vi "8255-led .vi"() -> ()   [LabVIEW 2010]
uses:
  <vilib>/LabVIEW Interface for Arduino/Type Defs/Pin Mode.ctl
  <vilib>/LabVIEW Interface for Arduino/LabVIEW Interface for Arduino.lvlib
panel:
  in  "Boolean":bool
  in  "OK Button":bool
  in  "Slide":dbl(slide) scale=0.0..1.0
  in  "stop":bool
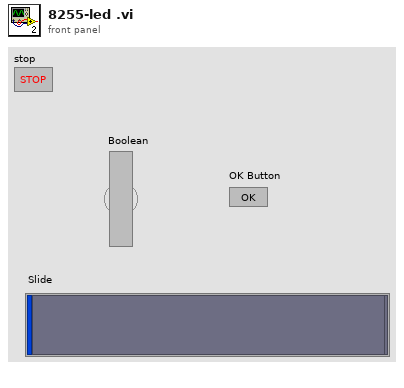
[diagram p1: front panel]
types:
  T1 = typedef "LabVIEW Interface for Arduino.lvlib/Arduino Resource.ctl" = cluster{"VISA resource":refnum<visa-resource-name>, "Board Type":T2, "Connection Type":enum8{"USB / Serial"}, "Bytes Per Packet (15)":u8}
  T2 = typedef "LabVIEW Interface for Arduino.lvlib/Board Type.ctl" = enum16{"Uno", "Dimuelanove w/Atmega 328", "Mega 2560"}
  T3 = typedef "LabVIEW Interface for Arduino.lvlib/Pin Mode.ctl" = enum8{"Input", "Output"}
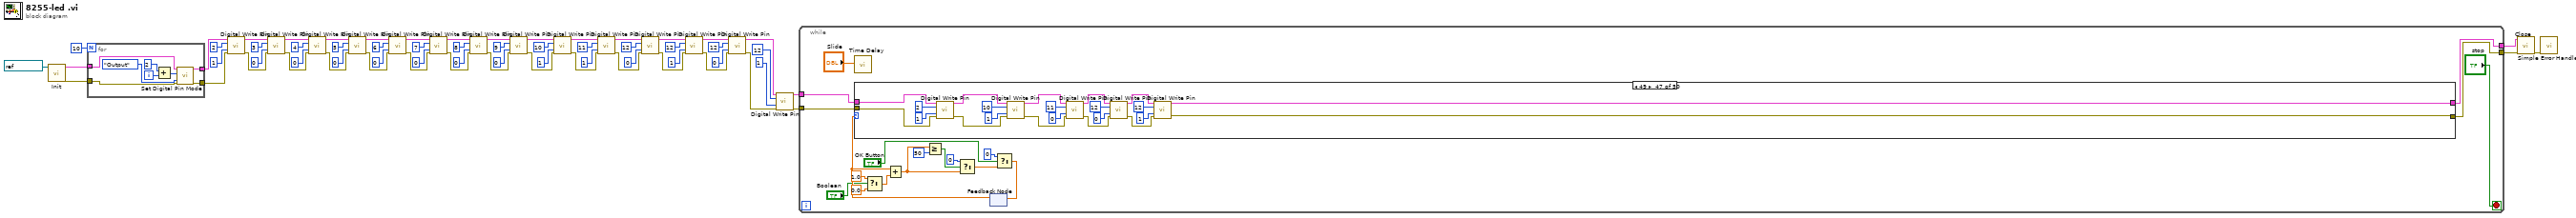
[diagram p0: block diagram]
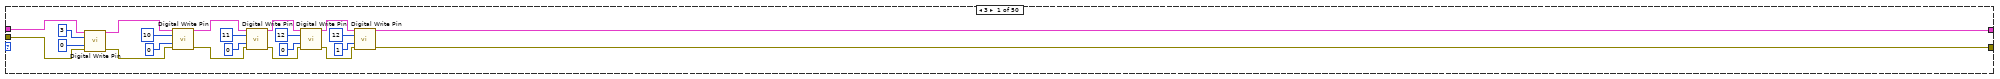
[diagram p2: hidden frame]
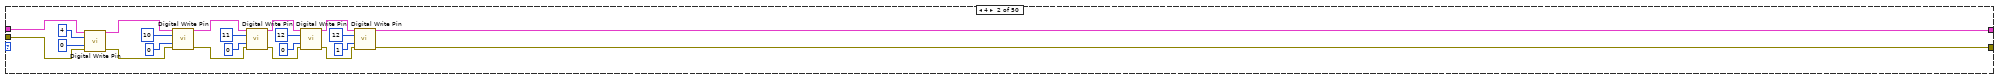
[diagram p3: hidden frame]
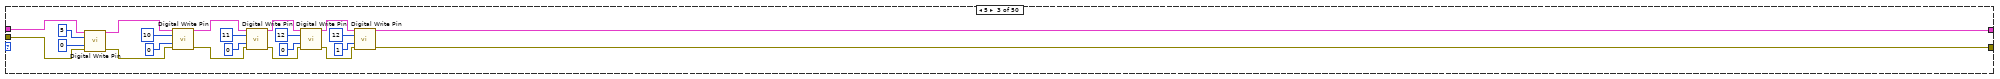
[diagram p4: hidden frame]
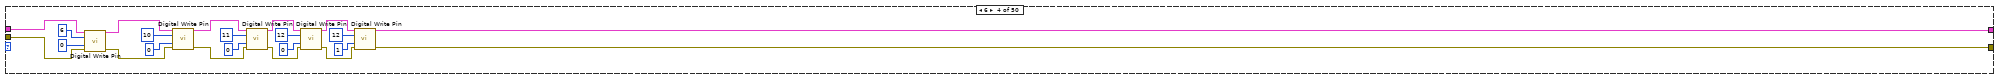
[diagram p5: hidden frame]
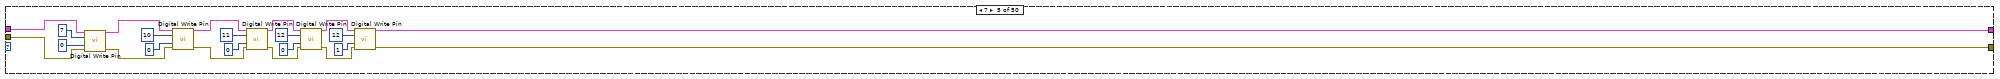
[diagram p6: hidden frame]
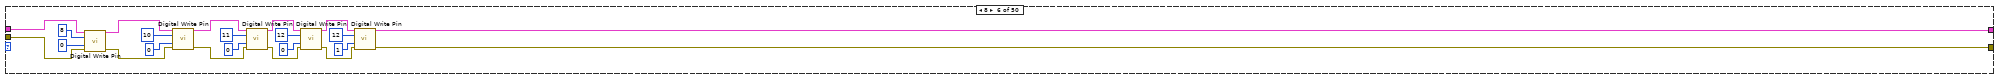
[diagram p7: hidden frame]
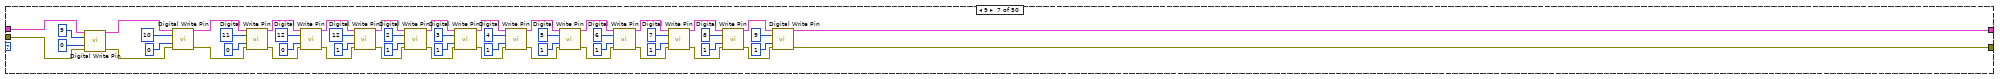
[diagram p8: hidden frame]
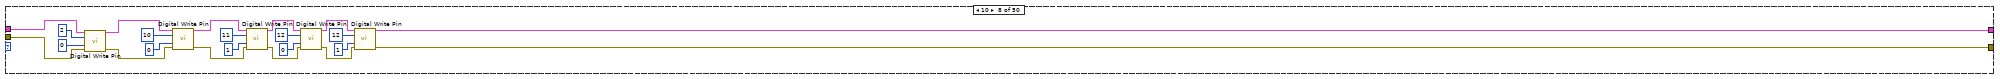
[diagram p9: hidden frame]
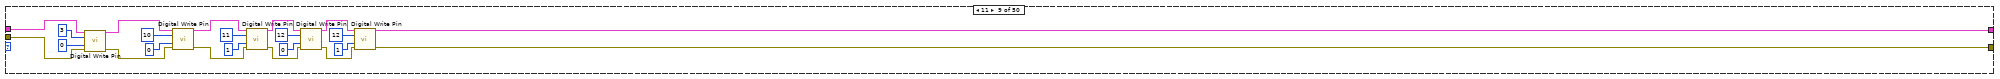
[diagram p10: hidden frame]
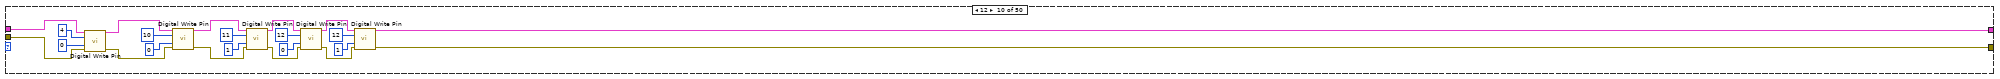
[diagram p11: hidden frame]
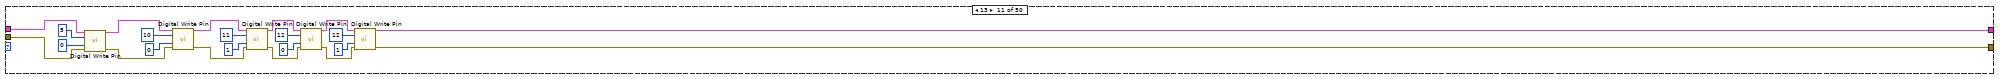
[diagram p12: hidden frame]
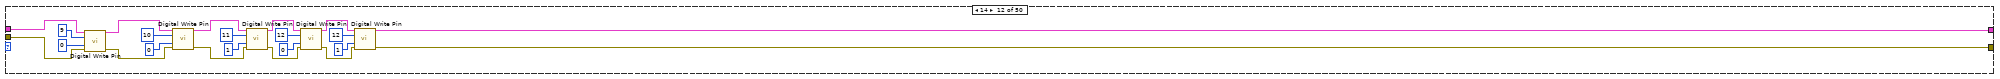
[diagram p13: hidden frame]
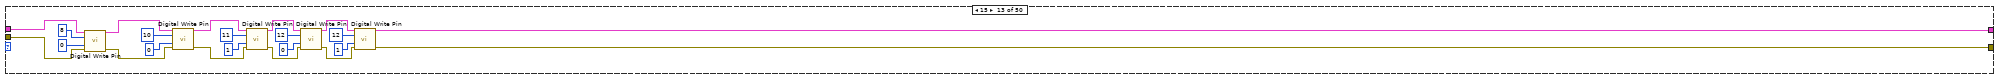
[diagram p14: hidden frame]
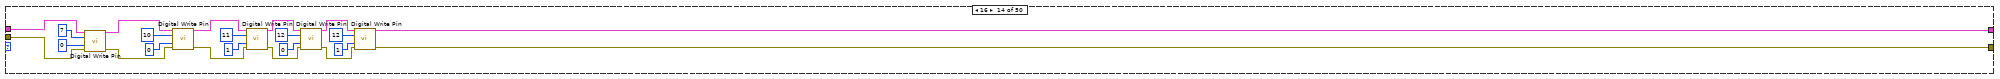
[diagram p15: hidden frame]
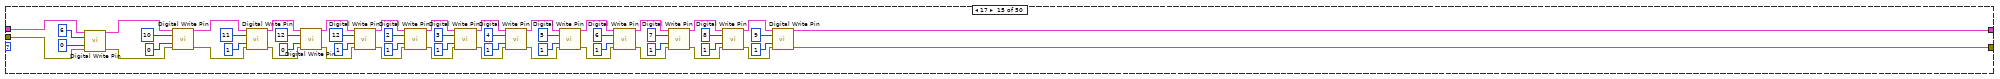
[diagram p16: hidden frame]
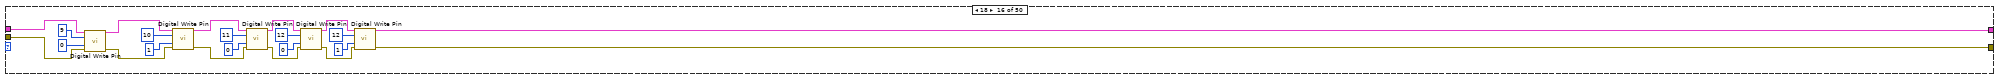
[diagram p17: hidden frame]
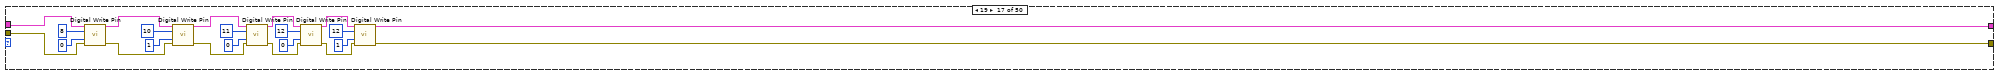
[diagram p18: hidden frame]
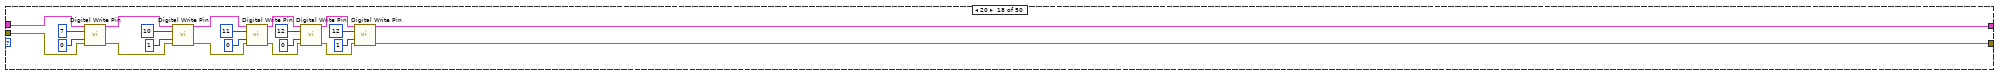
[diagram p19: hidden frame]
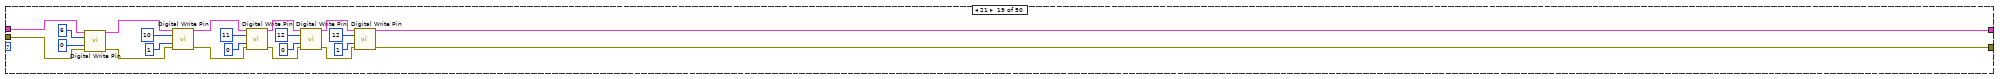
[diagram p20: hidden frame]
diagram:
  n1 = call <vilib>:"Init.vi"("VISA resource"=refnum<visa-resource-name> "COM35") -> ("Arduino Resource"=w64:T1, "error out"=w63:errorcluster)  [unwired: 17 in]
  n2 = for {
    N: 10 -> [_]
    tunnel: w64 -> [w73]
    tunnel: w63 -> [w72]
    tunnel: [w67] -> w61
    tunnel: [w66] -> w60
    i -> [w71]
    n3 = Add(x=2, y=w71) -> (x+y=w69:i32)
    n4 = call <vilib>:"Set Digital Pin Mode.vi"("Arduino Resource"=w73, "Digital I/O Pin"=w69, "Pin Mode (Input)"=Pin_Mode."Output", "error in"=w72) -> ("Arduino Resource"=w67:T1, "error out"=w66:errorcluster)  [unwired: 10 in]
  }
  n5 = call <vilib>:"Digital Write Pin.vi"("Arduino Resource"=w61, "Digital I/O Pin (0)"=u8 2, "Value (0)"=u8 1, "error in"=w60) -> ("Arduino Resource"=w59:T1, "error out"=w58:errorcluster)  [unwired: 10 in]
  n6 = call <vilib>:"Digital Write Pin.vi"("Arduino Resource"=w59, "Digital I/O Pin (0)"=u8 3, "Value (0)"=u8 0, "error in"=w58) -> ("Arduino Resource"=w57:T1, "error out"=w56:errorcluster)  [unwired: 10 in]
  n7 = call <vilib>:"Digital Write Pin.vi"("Arduino Resource"=w57, "Digital I/O Pin (0)"=u8 4, "Value (0)"=u8 0, "error in"=w56) -> ("Arduino Resource"=w55:T1, "error out"=w54:errorcluster)  [unwired: 10 in]
  n8 = call <vilib>:"Digital Write Pin.vi"("Arduino Resource"=w55, "Digital I/O Pin (0)"=u8 5, "Value (0)"=u8 0, "error in"=w54) -> ("Arduino Resource"=w53:T1, "error out"=w52:errorcluster)  [unwired: 10 in]
  n9 = call <vilib>:"Digital Write Pin.vi"("Arduino Resource"=w53, "Digital I/O Pin (0)"=u8 6, "Value (0)"=u8 0, "error in"=w52) -> ("Arduino Resource"=w51:T1, "error out"=w50:errorcluster)  [unwired: 10 in]
  n10 = call <vilib>:"Digital Write Pin.vi"("Arduino Resource"=w51, "Digital I/O Pin (0)"=u8 7, "Value (0)"=u8 0, "error in"=w50) -> ("Arduino Resource"=w49:T1, "error out"=w48:errorcluster)  [unwired: 10 in]
  n11 = call <vilib>:"Digital Write Pin.vi"("Arduino Resource"=w49, "Digital I/O Pin (0)"=u8 8, "Value (0)"=u8 0, "error in"=w48) -> ("Arduino Resource"=w47:T1, "error out"=w46:errorcluster)  [unwired: 10 in]
  n12 = call <vilib>:"Digital Write Pin.vi"("Arduino Resource"=w47, "Digital I/O Pin (0)"=u8 9, "Value (0)"=u8 0, "error in"=w46) -> ("Arduino Resource"=w45:T1, "error out"=w44:errorcluster)  [unwired: 10 in]
  n13 = call <vilib>:"Digital Write Pin.vi"("Arduino Resource"=w45, "Digital I/O Pin (0)"=u8 10, "Value (0)"=u8 1, "error in"=w44) -> ("Arduino Resource"=w43:T1, "error out"=w42:errorcluster)  [unwired: 10 in]
  n14 = call <vilib>:"Digital Write Pin.vi"("Arduino Resource"=w43, "Digital I/O Pin (0)"=u8 11, "Value (0)"=u8 1, "error in"=w42) -> ("Arduino Resource"=w21:T1, "error out"=w20:errorcluster)  [unwired: 10 in]
  n15 = call <vilib>:"Digital Write Pin.vi"("Arduino Resource"=w21, "Digital I/O Pin (0)"=u8 12, "Value (0)"=u8 0, "error in"=w20) -> ("Arduino Resource"=w11:T1, "error out"=w12:errorcluster)  [unwired: 10 in]
  n16 = call <vilib>:"Digital Write Pin.vi"("Arduino Resource"=w11, "Digital I/O Pin (0)"=u8 12, "Value (0)"=u8 1, "error in"=w12) -> ("Arduino Resource"=w10:T1, "error out"=w6:errorcluster)  [unwired: 10 in]
  n17 = call <vilib>:"Digital Write Pin.vi"("Arduino Resource"=w10, "Digital I/O Pin (0)"=u8 12, "Value (0)"=u8 0, "error in"=w6) -> ("Arduino Resource"=w9:T1, "error out"=w5:errorcluster)  [unwired: 10 in]
  n18 = call <vilib>:"Digital Write Pin.vi"("Arduino Resource"=w9, "Digital I/O Pin (0)"=u8 12, "Value (0)"=u8 1, "error in"=w5) -> ("Arduino Resource"=w8:T1, "error out"=w7:errorcluster)  [unwired: 10 in]
  n19 = while {
    tunnel: w8 -> [w88]
    tunnel: w7 -> [w87]
    tunnel: [w86] -> w3
    tunnel: [w85] -> w2
    stop <- "stop" stop-if-true
    n20 = call "Time Delay"("Delay Time (s)"="Slide") -> ()  [unwired: 10 in, 1 out]
    n21 = Select(t=1.0, s="Boolean", f=0.0) -> (s? t:f=w74:dbl)
    n22 = feedback #1() -> (w79:dbl)  [unwired: 1 in]
    n23 = case shown="49" w79 {
      tunnel: w88 -> [w95 w118 w140 w162 w184 w206 w260 w282 w304 w326 w358 w380 w402 w424 w478 w500 w522 w544 w566 w588 w610 w632 w654 w666 w692 w710 w732 w754 w776 w798 w820 w874 w896 w918 w940 w962 w984 w1006 w1028 w1086 w1104 w1126 w1148 w1170 w1192 w1214 w1236 w1261 w1278 w1426]
      tunnel: w87 -> [w96 w117 w139 w161 w183 w205 w259 w281 w303 w325 w357 w381 w401 w423 w477 w499 w521 w543 w565 w587 w609 w631 w653 w665 w691 w709 w731 w753 w775 w797 w819 w873 w895 w917 w939 w961 w983 w1005 w1027 w1085 w1103 w1125 w1147 w1169 w1191 w1213 w1235 w1260 w1277 w1425]
      tunnel: [w93 w115 w137 w159 w181 w203 w225 w279 w301 w323 w355 w377 w399 w421 w433 w487 w519 w541 w563 w585 w607 w629 w651 w663 w685 w707 w729 w752 w773 w795 w817 w871 w893 w915 w937 w959 w981 w1003 w1025 w1079 w1101 w1123 w1145 w1167 w1189 w1211 w1233 w1255 w1280 w1423] -> w86
      tunnel: [w94 w116 w138 w160 w182 w204 w226 w280 w302 w324 w356 w378 w400 w422 w434 w488 w520 w542 w564 w586 w608 w630 w652 w664 w686 w708 w730 w751 w774 w796 w818 w872 w894 w916 w938 w960 w982 w1004 w1026 w1080 w1102 w1124 w1146 w1168 w1190 w1212 w1234 w1256 w1281 w1424] -> w85
      frame 3 {
        n24 = call <vilib>:"Digital Write Pin.vi"("Arduino Resource"=w95, "Digital I/O Pin (0)"=u8 3, "Value (0)"=u8 0, "error in"=w96) -> ("Arduino Resource"=w98:T1, "error out"=w97:errorcluster)  [unwired: 10 in]
        n25 = call <vilib>:"Digital Write Pin.vi"("Arduino Resource"=w98, "Digital I/O Pin (0)"=u8 10, "Value (0)"=u8 0, "error in"=w97) -> ("Arduino Resource"=w106:T1, "error out"=w105:errorcluster)  [unwired: 10 in]
        n26 = call <vilib>:"Digital Write Pin.vi"("Arduino Resource"=w106, "Digital I/O Pin (0)"=u8 11, "Value (0)"=u8 0, "error in"=w105) -> ("Arduino Resource"=w107:T1, "error out"=w108:errorcluster)  [unwired: 10 in]
        n27 = call <vilib>:"Digital Write Pin.vi"("Arduino Resource"=w107, "Digital I/O Pin (0)"=u8 12, "Value (0)"=u8 0, "error in"=w108) -> ("Arduino Resource"=w110:T1, "error out"=w109:errorcluster)  [unwired: 10 in]
        n28 = call <vilib>:"Digital Write Pin.vi"("Arduino Resource"=w110, "Digital I/O Pin (0)"=u8 12, "Value (0)"=u8 1, "error in"=w109) -> ("Arduino Resource"=w94:T1, "error out"=w93:errorcluster)  [unwired: 10 in]
      }
      frame 4 {
        n29 = call <vilib>:"Digital Write Pin.vi"("Arduino Resource"=w118, "Digital I/O Pin (0)"=u8 4, "Value (0)"=u8 0, "error in"=w117) -> ("Arduino Resource"=w120:T1, "error out"=w119:errorcluster)  [unwired: 10 in]
        n30 = call <vilib>:"Digital Write Pin.vi"("Arduino Resource"=w120, "Digital I/O Pin (0)"=u8 10, "Value (0)"=u8 0, "error in"=w119) -> ("Arduino Resource"=w128:T1, "error out"=w127:errorcluster)  [unwired: 10 in]
        n31 = call <vilib>:"Digital Write Pin.vi"("Arduino Resource"=w128, "Digital I/O Pin (0)"=u8 11, "Value (0)"=u8 0, "error in"=w127) -> ("Arduino Resource"=w129:T1, "error out"=w130:errorcluster)  [unwired: 10 in]
        n32 = call <vilib>:"Digital Write Pin.vi"("Arduino Resource"=w129, "Digital I/O Pin (0)"=u8 12, "Value (0)"=u8 0, "error in"=w130) -> ("Arduino Resource"=w132:T1, "error out"=w131:errorcluster)  [unwired: 10 in]
        n33 = call <vilib>:"Digital Write Pin.vi"("Arduino Resource"=w132, "Digital I/O Pin (0)"=u8 12, "Value (0)"=u8 1, "error in"=w131) -> ("Arduino Resource"=w116:T1, "error out"=w115:errorcluster)  [unwired: 10 in]
      }
      frame 5 {
        n34 = call <vilib>:"Digital Write Pin.vi"("Arduino Resource"=w140, "Digital I/O Pin (0)"=u8 5, "Value (0)"=u8 0, "error in"=w139) -> ("Arduino Resource"=w142:T1, "error out"=w141:errorcluster)  [unwired: 10 in]
        n35 = call <vilib>:"Digital Write Pin.vi"("Arduino Resource"=w142, "Digital I/O Pin (0)"=u8 10, "Value (0)"=u8 0, "error in"=w141) -> ("Arduino Resource"=w150:T1, "error out"=w149:errorcluster)  [unwired: 10 in]
        n36 = call <vilib>:"Digital Write Pin.vi"("Arduino Resource"=w150, "Digital I/O Pin (0)"=u8 11, "Value (0)"=u8 0, "error in"=w149) -> ("Arduino Resource"=w151:T1, "error out"=w152:errorcluster)  [unwired: 10 in]
        n37 = call <vilib>:"Digital Write Pin.vi"("Arduino Resource"=w151, "Digital I/O Pin (0)"=u8 12, "Value (0)"=u8 0, "error in"=w152) -> ("Arduino Resource"=w154:T1, "error out"=w153:errorcluster)  [unwired: 10 in]
        n38 = call <vilib>:"Digital Write Pin.vi"("Arduino Resource"=w154, "Digital I/O Pin (0)"=u8 12, "Value (0)"=u8 1, "error in"=w153) -> ("Arduino Resource"=w138:T1, "error out"=w137:errorcluster)  [unwired: 10 in]
      }
      frame 6 {
        n39 = call <vilib>:"Digital Write Pin.vi"("Arduino Resource"=w162, "Digital I/O Pin (0)"=u8 6, "Value (0)"=u8 0, "error in"=w161) -> ("Arduino Resource"=w164:T1, "error out"=w163:errorcluster)  [unwired: 10 in]
        n40 = call <vilib>:"Digital Write Pin.vi"("Arduino Resource"=w164, "Digital I/O Pin (0)"=u8 10, "Value (0)"=u8 0, "error in"=w163) -> ("Arduino Resource"=w172:T1, "error out"=w171:errorcluster)  [unwired: 10 in]
        n41 = call <vilib>:"Digital Write Pin.vi"("Arduino Resource"=w172, "Digital I/O Pin (0)"=u8 11, "Value (0)"=u8 0, "error in"=w171) -> ("Arduino Resource"=w173:T1, "error out"=w174:errorcluster)  [unwired: 10 in]
        n42 = call <vilib>:"Digital Write Pin.vi"("Arduino Resource"=w173, "Digital I/O Pin (0)"=u8 12, "Value (0)"=u8 0, "error in"=w174) -> ("Arduino Resource"=w176:T1, "error out"=w175:errorcluster)  [unwired: 10 in]
        n43 = call <vilib>:"Digital Write Pin.vi"("Arduino Resource"=w176, "Digital I/O Pin (0)"=u8 12, "Value (0)"=u8 1, "error in"=w175) -> ("Arduino Resource"=w160:T1, "error out"=w159:errorcluster)  [unwired: 10 in]
      }
      frame 7 {
        n44 = call <vilib>:"Digital Write Pin.vi"("Arduino Resource"=w184, "Digital I/O Pin (0)"=u8 7, "Value (0)"=u8 0, "error in"=w183) -> ("Arduino Resource"=w186:T1, "error out"=w185:errorcluster)  [unwired: 10 in]
        n45 = call <vilib>:"Digital Write Pin.vi"("Arduino Resource"=w186, "Digital I/O Pin (0)"=u8 10, "Value (0)"=u8 0, "error in"=w185) -> ("Arduino Resource"=w194:T1, "error out"=w193:errorcluster)  [unwired: 10 in]
        n46 = call <vilib>:"Digital Write Pin.vi"("Arduino Resource"=w194, "Digital I/O Pin (0)"=u8 11, "Value (0)"=u8 0, "error in"=w193) -> ("Arduino Resource"=w195:T1, "error out"=w196:errorcluster)  [unwired: 10 in]
        n47 = call <vilib>:"Digital Write Pin.vi"("Arduino Resource"=w195, "Digital I/O Pin (0)"=u8 12, "Value (0)"=u8 0, "error in"=w196) -> ("Arduino Resource"=w198:T1, "error out"=w197:errorcluster)  [unwired: 10 in]
        n48 = call <vilib>:"Digital Write Pin.vi"("Arduino Resource"=w198, "Digital I/O Pin (0)"=u8 12, "Value (0)"=u8 1, "error in"=w197) -> ("Arduino Resource"=w182:T1, "error out"=w181:errorcluster)  [unwired: 10 in]
      }
      frame 8 {
        n49 = call <vilib>:"Digital Write Pin.vi"("Arduino Resource"=w206, "Digital I/O Pin (0)"=u8 8, "Value (0)"=u8 0, "error in"=w205) -> ("Arduino Resource"=w208:T1, "error out"=w207:errorcluster)  [unwired: 10 in]
        n50 = call <vilib>:"Digital Write Pin.vi"("Arduino Resource"=w208, "Digital I/O Pin (0)"=u8 10, "Value (0)"=u8 0, "error in"=w207) -> ("Arduino Resource"=w216:T1, "error out"=w215:errorcluster)  [unwired: 10 in]
        n51 = call <vilib>:"Digital Write Pin.vi"("Arduino Resource"=w216, "Digital I/O Pin (0)"=u8 11, "Value (0)"=u8 0, "error in"=w215) -> ("Arduino Resource"=w217:T1, "error out"=w218:errorcluster)  [unwired: 10 in]
        n52 = call <vilib>:"Digital Write Pin.vi"("Arduino Resource"=w217, "Digital I/O Pin (0)"=u8 12, "Value (0)"=u8 0, "error in"=w218) -> ("Arduino Resource"=w220:T1, "error out"=w219:errorcluster)  [unwired: 10 in]
        n53 = call <vilib>:"Digital Write Pin.vi"("Arduino Resource"=w220, "Digital I/O Pin (0)"=u8 12, "Value (0)"=u8 1, "error in"=w219) -> ("Arduino Resource"=w204:T1, "error out"=w203:errorcluster)  [unwired: 10 in]
      }
      frame 9 {
        n54 = call <vilib>:"Digital Write Pin.vi"("Arduino Resource"=w260, "Digital I/O Pin (0)"=u8 9, "Value (0)"=u8 0, "error in"=w259) -> ("Arduino Resource"=w262:T1, "error out"=w261:errorcluster)  [unwired: 10 in]
        n55 = call <vilib>:"Digital Write Pin.vi"("Arduino Resource"=w262, "Digital I/O Pin (0)"=u8 10, "Value (0)"=u8 0, "error in"=w261) -> ("Arduino Resource"=w270:T1, "error out"=w269:errorcluster)  [unwired: 10 in]
        n56 = call <vilib>:"Digital Write Pin.vi"("Arduino Resource"=w270, "Digital I/O Pin (0)"=u8 11, "Value (0)"=u8 0, "error in"=w269) -> ("Arduino Resource"=w271:T1, "error out"=w272:errorcluster)  [unwired: 10 in]
        n57 = call <vilib>:"Digital Write Pin.vi"("Arduino Resource"=w271, "Digital I/O Pin (0)"=u8 12, "Value (0)"=u8 0, "error in"=w272) -> ("Arduino Resource"=w274:T1, "error out"=w273:errorcluster)  [unwired: 10 in]
        n58 = call <vilib>:"Digital Write Pin.vi"("Arduino Resource"=w274, "Digital I/O Pin (0)"=u8 12, "Value (0)"=u8 1, "error in"=w273) -> ("Arduino Resource"=w228:T1, "error out"=w227:errorcluster)  [unwired: 10 in]
        n59 = call <vilib>:"Digital Write Pin.vi"("Arduino Resource"=w228, "Digital I/O Pin (0)"=u8 2, "Value (0)"=u8 1, "error in"=w227) -> ("Arduino Resource"=w258:T1, "error out"=w257:errorcluster)  [unwired: 10 in]
        n60 = call <vilib>:"Digital Write Pin.vi"("Arduino Resource"=w258, "Digital I/O Pin (0)"=u8 3, "Value (0)"=u8 1, "error in"=w257) -> ("Arduino Resource"=w256:T1, "error out"=w255:errorcluster)  [unwired: 10 in]
        n61 = call <vilib>:"Digital Write Pin.vi"("Arduino Resource"=w256, "Digital I/O Pin (0)"=u8 4, "Value (0)"=u8 1, "error in"=w255) -> ("Arduino Resource"=w254:T1, "error out"=w253:errorcluster)  [unwired: 10 in]
        n62 = call <vilib>:"Digital Write Pin.vi"("Arduino Resource"=w254, "Digital I/O Pin (0)"=u8 5, "Value (0)"=u8 1, "error in"=w253) -> ("Arduino Resource"=w252:T1, "error out"=w251:errorcluster)  [unwired: 10 in]
        n63 = call <vilib>:"Digital Write Pin.vi"("Arduino Resource"=w252, "Digital I/O Pin (0)"=u8 6, "Value (0)"=u8 1, "error in"=w251) -> ("Arduino Resource"=w250:T1, "error out"=w249:errorcluster)  [unwired: 10 in]
        n64 = call <vilib>:"Digital Write Pin.vi"("Arduino Resource"=w250, "Digital I/O Pin (0)"=u8 7, "Value (0)"=u8 1, "error in"=w249) -> ("Arduino Resource"=w248:T1, "error out"=w247:errorcluster)  [unwired: 10 in]
        n65 = call <vilib>:"Digital Write Pin.vi"("Arduino Resource"=w248, "Digital I/O Pin (0)"=u8 8, "Value (0)"=u8 1, "error in"=w247) -> ("Arduino Resource"=w246:T1, "error out"=w245:errorcluster)  [unwired: 10 in]
        n66 = call <vilib>:"Digital Write Pin.vi"("Arduino Resource"=w246, "Digital I/O Pin (0)"=u8 9, "Value (0)"=u8 1, "error in"=w245) -> ("Arduino Resource"=w226:T1, "error out"=w225:errorcluster)  [unwired: 10 in]
      }
      frame 10 {
        n67 = call <vilib>:"Digital Write Pin.vi"("Arduino Resource"=w282, "Digital I/O Pin (0)"=u8 2, "Value (0)"=u8 0, "error in"=w281) -> ("Arduino Resource"=w284:T1, "error out"=w283:errorcluster)  [unwired: 10 in]
        n68 = call <vilib>:"Digital Write Pin.vi"("Arduino Resource"=w284, "Digital I/O Pin (0)"=u8 10, "Value (0)"=u8 0, "error in"=w283) -> ("Arduino Resource"=w292:T1, "error out"=w291:errorcluster)  [unwired: 10 in]
        n69 = call <vilib>:"Digital Write Pin.vi"("Arduino Resource"=w292, "Digital I/O Pin (0)"=u8 11, "Value (0)"=u8 1, "error in"=w291) -> ("Arduino Resource"=w293:T1, "error out"=w294:errorcluster)  [unwired: 10 in]
        n70 = call <vilib>:"Digital Write Pin.vi"("Arduino Resource"=w293, "Digital I/O Pin (0)"=u8 12, "Value (0)"=u8 0, "error in"=w294) -> ("Arduino Resource"=w296:T1, "error out"=w295:errorcluster)  [unwired: 10 in]
        n71 = call <vilib>:"Digital Write Pin.vi"("Arduino Resource"=w296, "Digital I/O Pin (0)"=u8 12, "Value (0)"=u8 1, "error in"=w295) -> ("Arduino Resource"=w280:T1, "error out"=w279:errorcluster)  [unwired: 10 in]
      }
      frame 11 {
        n72 = call <vilib>:"Digital Write Pin.vi"("Arduino Resource"=w304, "Digital I/O Pin (0)"=u8 3, "Value (0)"=u8 0, "error in"=w303) -> ("Arduino Resource"=w306:T1, "error out"=w305:errorcluster)  [unwired: 10 in]
        n73 = call <vilib>:"Digital Write Pin.vi"("Arduino Resource"=w306, "Digital I/O Pin (0)"=u8 10, "Value (0)"=u8 0, "error in"=w305) -> ("Arduino Resource"=w314:T1, "error out"=w313:errorcluster)  [unwired: 10 in]
        n74 = call <vilib>:"Digital Write Pin.vi"("Arduino Resource"=w314, "Digital I/O Pin (0)"=u8 11, "Value (0)"=u8 1, "error in"=w313) -> ("Arduino Resource"=w315:T1, "error out"=w316:errorcluster)  [unwired: 10 in]
        n75 = call <vilib>:"Digital Write Pin.vi"("Arduino Resource"=w315, "Digital I/O Pin (0)"=u8 12, "Value (0)"=u8 0, "error in"=w316) -> ("Arduino Resource"=w318:T1, "error out"=w317:errorcluster)  [unwired: 10 in]
        n76 = call <vilib>:"Digital Write Pin.vi"("Arduino Resource"=w318, "Digital I/O Pin (0)"=u8 12, "Value (0)"=u8 1, "error in"=w317) -> ("Arduino Resource"=w302:T1, "error out"=w301:errorcluster)  [unwired: 10 in]
      }
      frame 12 {
        n77 = call <vilib>:"Digital Write Pin.vi"("Arduino Resource"=w326, "Digital I/O Pin (0)"=u8 4, "Value (0)"=u8 0, "error in"=w325) -> ("Arduino Resource"=w328:T1, "error out"=w327:errorcluster)  [unwired: 10 in]
        n78 = call <vilib>:"Digital Write Pin.vi"("Arduino Resource"=w328, "Digital I/O Pin (0)"=u8 10, "Value (0)"=u8 0, "error in"=w327) -> ("Arduino Resource"=w336:T1, "error out"=w335:errorcluster)  [unwired: 10 in]
        n79 = call <vilib>:"Digital Write Pin.vi"("Arduino Resource"=w336, "Digital I/O Pin (0)"=u8 11, "Value (0)"=u8 1, "error in"=w335) -> ("Arduino Resource"=w337:T1, "error out"=w338:errorcluster)  [unwired: 10 in]
        n80 = call <vilib>:"Digital Write Pin.vi"("Arduino Resource"=w337, "Digital I/O Pin (0)"=u8 12, "Value (0)"=u8 0, "error in"=w338) -> ("Arduino Resource"=w340:T1, "error out"=w339:errorcluster)  [unwired: 10 in]
        n81 = call <vilib>:"Digital Write Pin.vi"("Arduino Resource"=w340, "Digital I/O Pin (0)"=u8 12, "Value (0)"=u8 1, "error in"=w339) -> ("Arduino Resource"=w324:T1, "error out"=w323:errorcluster)  [unwired: 10 in]
      }
      frame 13 {
        n82 = call <vilib>:"Digital Write Pin.vi"("Arduino Resource"=w358, "Digital I/O Pin (0)"=u8 5, "Value (0)"=u8 0, "error in"=w357) -> ("Arduino Resource"=w348:T1, "error out"=w347:errorcluster)  [unwired: 10 in]
        n83 = call <vilib>:"Digital Write Pin.vi"("Arduino Resource"=w348, "Digital I/O Pin (0)"=u8 10, "Value (0)"=u8 0, "error in"=w347) -> ("Arduino Resource"=w354:T1, "error out"=w353:errorcluster)  [unwired: 10 in]
        n84 = call <vilib>:"Digital Write Pin.vi"("Arduino Resource"=w354, "Digital I/O Pin (0)"=u8 11, "Value (0)"=u8 1, "error in"=w353) -> ("Arduino Resource"=w346:T1, "error out"=w345:errorcluster)  [unwired: 10 in]
        n85 = call <vilib>:"Digital Write Pin.vi"("Arduino Resource"=w346, "Digital I/O Pin (0)"=u8 12, "Value (0)"=u8 0, "error in"=w345) -> ("Arduino Resource"=w362:T1, "error out"=w361:errorcluster)  [unwired: 10 in]
        n86 = call <vilib>:"Digital Write Pin.vi"("Arduino Resource"=w362, "Digital I/O Pin (0)"=u8 12, "Value (0)"=u8 1, "error in"=w361) -> ("Arduino Resource"=w356:T1, "error out"=w355:errorcluster)  [unwired: 10 in]
      }
      frame 14 {
        n87 = call <vilib>:"Digital Write Pin.vi"("Arduino Resource"=w380, "Digital I/O Pin (0)"=u8 9, "Value (0)"=u8 0, "error in"=w381) -> ("Arduino Resource"=w370:T1, "error out"=w369:errorcluster)  [unwired: 10 in]
        n88 = call <vilib>:"Digital Write Pin.vi"("Arduino Resource"=w370, "Digital I/O Pin (0)"=u8 10, "Value (0)"=u8 0, "error in"=w369) -> ("Arduino Resource"=w376:T1, "error out"=w375:errorcluster)  [unwired: 10 in]
        n89 = call <vilib>:"Digital Write Pin.vi"("Arduino Resource"=w376, "Digital I/O Pin (0)"=u8 11, "Value (0)"=u8 1, "error in"=w375) -> ("Arduino Resource"=w368:T1, "error out"=w367:errorcluster)  [unwired: 10 in]
        n90 = call <vilib>:"Digital Write Pin.vi"("Arduino Resource"=w368, "Digital I/O Pin (0)"=u8 12, "Value (0)"=u8 0, "error in"=w367) -> ("Arduino Resource"=w379:T1, "error out"=w384:errorcluster)  [unwired: 10 in]
        n91 = call <vilib>:"Digital Write Pin.vi"("Arduino Resource"=w379, "Digital I/O Pin (0)"=u8 12, "Value (0)"=u8 1, "error in"=w384) -> ("Arduino Resource"=w378:T1, "error out"=w377:errorcluster)  [unwired: 10 in]
      }
      frame 15 {
        n92 = call <vilib>:"Digital Write Pin.vi"("Arduino Resource"=w402, "Digital I/O Pin (0)"=u8 8, "Value (0)"=u8 0, "error in"=w401) -> ("Arduino Resource"=w392:T1, "error out"=w391:errorcluster)  [unwired: 10 in]
        n93 = call <vilib>:"Digital Write Pin.vi"("Arduino Resource"=w392, "Digital I/O Pin (0)"=u8 10, "Value (0)"=u8 0, "error in"=w391) -> ("Arduino Resource"=w398:T1, "error out"=w397:errorcluster)  [unwired: 10 in]
        n94 = call <vilib>:"Digital Write Pin.vi"("Arduino Resource"=w398, "Digital I/O Pin (0)"=u8 11, "Value (0)"=u8 1, "error in"=w397) -> ("Arduino Resource"=w389:T1, "error out"=w390:errorcluster)  [unwired: 10 in]
        n95 = call <vilib>:"Digital Write Pin.vi"("Arduino Resource"=w389, "Digital I/O Pin (0)"=u8 12, "Value (0)"=u8 0, "error in"=w390) -> ("Arduino Resource"=w406:T1, "error out"=w405:errorcluster)  [unwired: 10 in]
        n96 = call <vilib>:"Digital Write Pin.vi"("Arduino Resource"=w406, "Digital I/O Pin (0)"=u8 12, "Value (0)"=u8 1, "error in"=w405) -> ("Arduino Resource"=w400:T1, "error out"=w399:errorcluster)  [unwired: 10 in]
      }
      frame 16 {
        n97 = call <vilib>:"Digital Write Pin.vi"("Arduino Resource"=w424, "Digital I/O Pin (0)"=u8 7, "Value (0)"=u8 0, "error in"=w423) -> ("Arduino Resource"=w414:T1, "error out"=w413:errorcluster)  [unwired: 10 in]
        n98 = call <vilib>:"Digital Write Pin.vi"("Arduino Resource"=w414, "Digital I/O Pin (0)"=u8 10, "Value (0)"=u8 0, "error in"=w413) -> ("Arduino Resource"=w420:T1, "error out"=w419:errorcluster)  [unwired: 10 in]
        n99 = call <vilib>:"Digital Write Pin.vi"("Arduino Resource"=w420, "Digital I/O Pin (0)"=u8 11, "Value (0)"=u8 1, "error in"=w419) -> ("Arduino Resource"=w412:T1, "error out"=w411:errorcluster)  [unwired: 10 in]
        n100 = call <vilib>:"Digital Write Pin.vi"("Arduino Resource"=w412, "Digital I/O Pin (0)"=u8 12, "Value (0)"=u8 0, "error in"=w411) -> ("Arduino Resource"=w428:T1, "error out"=w427:errorcluster)  [unwired: 10 in]
        n101 = call <vilib>:"Digital Write Pin.vi"("Arduino Resource"=w428, "Digital I/O Pin (0)"=u8 12, "Value (0)"=u8 1, "error in"=w427) -> ("Arduino Resource"=w422:T1, "error out"=w421:errorcluster)  [unwired: 10 in]
      }
      frame 17 {
        n102 = call <vilib>:"Digital Write Pin.vi"("Arduino Resource"=w478, "Digital I/O Pin (0)"=u8 6, "Value (0)"=u8 0, "error in"=w477) -> ("Arduino Resource"=w470:T1, "error out"=w469:errorcluster)  [unwired: 10 in]
        n103 = call <vilib>:"Digital Write Pin.vi"("Arduino Resource"=w470, "Digital I/O Pin (0)"=u8 10, "Value (0)"=u8 0, "error in"=w469) -> ("Arduino Resource"=w476:T1, "error out"=w475:errorcluster)  [unwired: 10 in]
        n104 = call <vilib>:"Digital Write Pin.vi"("Arduino Resource"=w476, "Digital I/O Pin (0)"=u8 11, "Value (0)"=u8 1, "error in"=w475) -> ("Arduino Resource"=w468:T1, "error out"=w467:errorcluster)  [unwired: 10 in]
        n105 = call <vilib>:"Digital Write Pin.vi"("Arduino Resource"=w468, "Digital I/O Pin (0)"=u8 12, "Value (0)"=u8 0, "error in"=w467) -> ("Arduino Resource"=w482:T1, "error out"=w481:errorcluster)  [unwired: 10 in]
        n106 = call <vilib>:"Digital Write Pin.vi"("Arduino Resource"=w482, "Digital I/O Pin (0)"=u8 12, "Value (0)"=u8 1, "error in"=w481) -> ("Arduino Resource"=w436:T1, "error out"=w435:errorcluster)  [unwired: 10 in]
        n107 = call <vilib>:"Digital Write Pin.vi"("Arduino Resource"=w436, "Digital I/O Pin (0)"=u8 2, "Value (0)"=u8 1, "error in"=w435) -> ("Arduino Resource"=w466:T1, "error out"=w465:errorcluster)  [unwired: 10 in]
        n108 = call <vilib>:"Digital Write Pin.vi"("Arduino Resource"=w466, "Digital I/O Pin (0)"=u8 3, "Value (0)"=u8 1, "error in"=w465) -> ("Arduino Resource"=w464:T1, "error out"=w463:errorcluster)  [unwired: 10 in]
        n109 = call <vilib>:"Digital Write Pin.vi"("Arduino Resource"=w464, "Digital I/O Pin (0)"=u8 4, "Value (0)"=u8 1, "error in"=w463) -> ("Arduino Resource"=w462:T1, "error out"=w461:errorcluster)  [unwired: 10 in]
        n110 = call <vilib>:"Digital Write Pin.vi"("Arduino Resource"=w462, "Digital I/O Pin (0)"=u8 5, "Value (0)"=u8 1, "error in"=w461) -> ("Arduino Resource"=w460:T1, "error out"=w459:errorcluster)  [unwired: 10 in]
        n111 = call <vilib>:"Digital Write Pin.vi"("Arduino Resource"=w460, "Digital I/O Pin (0)"=u8 6, "Value (0)"=u8 1, "error in"=w459) -> ("Arduino Resource"=w458:T1, "error out"=w457:errorcluster)  [unwired: 10 in]
        n112 = call <vilib>:"Digital Write Pin.vi"("Arduino Resource"=w458, "Digital I/O Pin (0)"=u8 7, "Value (0)"=u8 1, "error in"=w457) -> ("Arduino Resource"=w456:T1, "error out"=w455:errorcluster)  [unwired: 10 in]
        n113 = call <vilib>:"Digital Write Pin.vi"("Arduino Resource"=w456, "Digital I/O Pin (0)"=u8 8, "Value (0)"=u8 1, "error in"=w455) -> ("Arduino Resource"=w454:T1, "error out"=w453:errorcluster)  [unwired: 10 in]
        n114 = call <vilib>:"Digital Write Pin.vi"("Arduino Resource"=w454, "Digital I/O Pin (0)"=u8 9, "Value (0)"=u8 1, "error in"=w453) -> ("Arduino Resource"=w434:T1, "error out"=w433:errorcluster)  [unwired: 10 in]
      }
      frame 18 {
        n115 = call <vilib>:"Digital Write Pin.vi"("Arduino Resource"=w500, "Digital I/O Pin (0)"=u8 9, "Value (0)"=u8 0, "error in"=w499) -> ("Arduino Resource"=w493:T1, "error out"=w492:errorcluster)  [unwired: 10 in]
        n116 = call <vilib>:"Digital Write Pin.vi"("Arduino Resource"=w493, "Digital I/O Pin (0)"=u8 10, "Value (0)"=u8 1, "error in"=w492) -> ("Arduino Resource"=w491:T1, "error out"=w498:errorcluster)  [unwired: 10 in]
        n117 = call <vilib>:"Digital Write Pin.vi"("Arduino Resource"=w491, "Digital I/O Pin (0)"=u8 11, "Value (0)"=u8 0, "error in"=w498) -> ("Arduino Resource"=w490:T1, "error out"=w489:errorcluster)  [unwired: 10 in]
        n118 = call <vilib>:"Digital Write Pin.vi"("Arduino Resource"=w490, "Digital I/O Pin (0)"=u8 12, "Value (0)"=u8 0, "error in"=w489) -> ("Arduino Resource"=w504:T1, "error out"=w503:errorcluster)  [unwired: 10 in]
        n119 = call <vilib>:"Digital Write Pin.vi"("Arduino Resource"=w504, "Digital I/O Pin (0)"=u8 12, "Value (0)"=u8 1, "error in"=w503) -> ("Arduino Resource"=w488:T1, "error out"=w487:errorcluster)  [unwired: 10 in]
      }
      frame 19 {
        n120 = call <vilib>:"Digital Write Pin.vi"("Arduino Resource"=w522, "Digital I/O Pin (0)"=u8 8, "Value (0)"=u8 0, "error in"=w521) -> ("Arduino Resource"=w512:T1, "error out"=w511:errorcluster)  [unwired: 10 in]
        n121 = call <vilib>:"Digital Write Pin.vi"("Arduino Resource"=w512, "Digital I/O Pin (0)"=u8 10, "Value (0)"=u8 1, "error in"=w511) -> ("Arduino Resource"=w513:T1, "error out"=w518:errorcluster)  [unwired: 10 in]
        n122 = call <vilib>:"Digital Write Pin.vi"("Arduino Resource"=w513, "Digital I/O Pin (0)"=u8 11, "Value (0)"=u8 0, "error in"=w518) -> ("Arduino Resource"=w510:T1, "error out"=w509:errorcluster)  [unwired: 10 in]
        n123 = call <vilib>:"Digital Write Pin.vi"("Arduino Resource"=w510, "Digital I/O Pin (0)"=u8 12, "Value (0)"=u8 0, "error in"=w509) -> ("Arduino Resource"=w526:T1, "error out"=w525:errorcluster)  [unwired: 10 in]
        n124 = call <vilib>:"Digital Write Pin.vi"("Arduino Resource"=w526, "Digital I/O Pin (0)"=u8 12, "Value (0)"=u8 1, "error in"=w525) -> ("Arduino Resource"=w520:T1, "error out"=w519:errorcluster)  [unwired: 10 in]
      }
      frame 20 {
        n125 = call <vilib>:"Digital Write Pin.vi"("Arduino Resource"=w544, "Digital I/O Pin (0)"=u8 7, "Value (0)"=u8 0, "error in"=w543) -> ("Arduino Resource"=w534:T1, "error out"=w533:errorcluster)  [unwired: 10 in]
        n126 = call <vilib>:"Digital Write Pin.vi"("Arduino Resource"=w534, "Digital I/O Pin (0)"=u8 10, "Value (0)"=u8 1, "error in"=w533) -> ("Arduino Resource"=w535:T1, "error out"=w540:errorcluster)  [unwired: 10 in]
        n127 = call <vilib>:"Digital Write Pin.vi"("Arduino Resource"=w535, "Digital I/O Pin (0)"=u8 11, "Value (0)"=u8 0, "error in"=w540) -> ("Arduino Resource"=w532:T1, "error out"=w531:errorcluster)  [unwired: 10 in]
        n128 = call <vilib>:"Digital Write Pin.vi"("Arduino Resource"=w532, "Digital I/O Pin (0)"=u8 12, "Value (0)"=u8 0, "error in"=w531) -> ("Arduino Resource"=w548:T1, "error out"=w547:errorcluster)  [unwired: 10 in]
        n129 = call <vilib>:"Digital Write Pin.vi"("Arduino Resource"=w548, "Digital I/O Pin (0)"=u8 12, "Value (0)"=u8 1, "error in"=w547) -> ("Arduino Resource"=w542:T1, "error out"=w541:errorcluster)  [unwired: 10 in]
      }
      frame 21 {
        n130 = call <vilib>:"Digital Write Pin.vi"("Arduino Resource"=w566, "Digital I/O Pin (0)"=u8 6, "Value (0)"=u8 0, "error in"=w565) -> ("Arduino Resource"=w556:T1, "error out"=w555:errorcluster)  [unwired: 10 in]
        n131 = call <vilib>:"Digital Write Pin.vi"("Arduino Resource"=w556, "Digital I/O Pin (0)"=u8 10, "Value (0)"=u8 1, "error in"=w555) -> ("Arduino Resource"=w557:T1, "error out"=w562:errorcluster)  [unwired: 10 in]
        n132 = call <vilib>:"Digital Write Pin.vi"("Arduino Resource"=w557, "Digital I/O Pin (0)"=u8 11, "Value (0)"=u8 0, "error in"=w562) -> ("Arduino Resource"=w554:T1, "error out"=w553:errorcluster)  [unwired: 10 in]
        n133 = call <vilib>:"Digital Write Pin.vi"("Arduino Resource"=w554, "Digital I/O Pin (0)"=u8 12, "Value (0)"=u8 0, "error in"=w553) -> ("Arduino Resource"=w570:T1, "error out"=w569:errorcluster)  [unwired: 10 in]
        n134 = call <vilib>:"Digital Write Pin.vi"("Arduino Resource"=w570, "Digital I/O Pin (0)"=u8 12, "Value (0)"=u8 1, "error in"=w569) -> ("Arduino Resource"=w564:T1, "error out"=w563:errorcluster)  [unwired: 10 in]
      }
      frame 22 {
        n135 = call <vilib>:"Digital Write Pin.vi"("Arduino Resource"=w588, "Digital I/O Pin (0)"=u8 5, "Value (0)"=u8 0, "error in"=w587) -> ("Arduino Resource"=w578:T1, "error out"=w577:errorcluster)  [unwired: 10 in]
        n136 = call <vilib>:"Digital Write Pin.vi"("Arduino Resource"=w578, "Digital I/O Pin (0)"=u8 10, "Value (0)"=u8 1, "error in"=w577) -> ("Arduino Resource"=w579:T1, "error out"=w584:errorcluster)  [unwired: 10 in]
        n137 = call <vilib>:"Digital Write Pin.vi"("Arduino Resource"=w579, "Digital I/O Pin (0)"=u8 11, "Value (0)"=u8 0, "error in"=w584) -> ("Arduino Resource"=w576:T1, "error out"=w575:errorcluster)  [unwired: 10 in]
        n138 = call <vilib>:"Digital Write Pin.vi"("Arduino Resource"=w576, "Digital I/O Pin (0)"=u8 12, "Value (0)"=u8 0, "error in"=w575) -> ("Arduino Resource"=w592:T1, "error out"=w591:errorcluster)  [unwired: 10 in]
        n139 = call <vilib>:"Digital Write Pin.vi"("Arduino Resource"=w592, "Digital I/O Pin (0)"=u8 12, "Value (0)"=u8 1, "error in"=w591) -> ("Arduino Resource"=w586:T1, "error out"=w585:errorcluster)  [unwired: 10 in]
      }
      frame 23 {
        n140 = call <vilib>:"Digital Write Pin.vi"("Arduino Resource"=w610, "Digital I/O Pin (0)"=u8 4, "Value (0)"=u8 0, "error in"=w609) -> ("Arduino Resource"=w600:T1, "error out"=w599:errorcluster)  [unwired: 10 in]
        n141 = call <vilib>:"Digital Write Pin.vi"("Arduino Resource"=w600, "Digital I/O Pin (0)"=u8 10, "Value (0)"=u8 1, "error in"=w599) -> ("Arduino Resource"=w601:T1, "error out"=w606:errorcluster)  [unwired: 10 in]
        n142 = call <vilib>:"Digital Write Pin.vi"("Arduino Resource"=w601, "Digital I/O Pin (0)"=u8 11, "Value (0)"=u8 0, "error in"=w606) -> ("Arduino Resource"=w598:T1, "error out"=w597:errorcluster)  [unwired: 10 in]
        n143 = call <vilib>:"Digital Write Pin.vi"("Arduino Resource"=w598, "Digital I/O Pin (0)"=u8 12, "Value (0)"=u8 0, "error in"=w597) -> ("Arduino Resource"=w614:T1, "error out"=w613:errorcluster)  [unwired: 10 in]
        n144 = call <vilib>:"Digital Write Pin.vi"("Arduino Resource"=w614, "Digital I/O Pin (0)"=u8 12, "Value (0)"=u8 1, "error in"=w613) -> ("Arduino Resource"=w608:T1, "error out"=w607:errorcluster)  [unwired: 10 in]
      }
      frame 24 {
        n145 = call <vilib>:"Digital Write Pin.vi"("Arduino Resource"=w632, "Digital I/O Pin (0)"=u8 3, "Value (0)"=u8 0, "error in"=w631) -> ("Arduino Resource"=w622:T1, "error out"=w621:errorcluster)  [unwired: 10 in]
        n146 = call <vilib>:"Digital Write Pin.vi"("Arduino Resource"=w622, "Digital I/O Pin (0)"=u8 10, "Value (0)"=u8 1, "error in"=w621) -> ("Arduino Resource"=w623:T1, "error out"=w628:errorcluster)  [unwired: 10 in]
        n147 = call <vilib>:"Digital Write Pin.vi"("Arduino Resource"=w623, "Digital I/O Pin (0)"=u8 11, "Value (0)"=u8 0, "error in"=w628) -> ("Arduino Resource"=w620:T1, "error out"=w619:errorcluster)  [unwired: 10 in]
        n148 = call <vilib>:"Digital Write Pin.vi"("Arduino Resource"=w620, "Digital I/O Pin (0)"=u8 12, "Value (0)"=u8 0, "error in"=w619) -> ("Arduino Resource"=w636:T1, "error out"=w635:errorcluster)  [unwired: 10 in]
        n149 = call <vilib>:"Digital Write Pin.vi"("Arduino Resource"=w636, "Digital I/O Pin (0)"=u8 12, "Value (0)"=u8 1, "error in"=w635) -> ("Arduino Resource"=w630:T1, "error out"=w629:errorcluster)  [unwired: 10 in]
      }
      frame 25 {
        n150 = call <vilib>:"Digital Write Pin.vi"("Arduino Resource"=w654, "Digital I/O Pin (0)"=u8 2, "Value (0)"=u8 0, "error in"=w653) -> ("Arduino Resource"=w644:T1, "error out"=w643:errorcluster)  [unwired: 10 in]
        n151 = call <vilib>:"Digital Write Pin.vi"("Arduino Resource"=w644, "Digital I/O Pin (0)"=u8 10, "Value (0)"=u8 1, "error in"=w643) -> ("Arduino Resource"=w645:T1, "error out"=w650:errorcluster)  [unwired: 10 in]
        n152 = call <vilib>:"Digital Write Pin.vi"("Arduino Resource"=w645, "Digital I/O Pin (0)"=u8 11, "Value (0)"=u8 0, "error in"=w650) -> ("Arduino Resource"=w642:T1, "error out"=w641:errorcluster)  [unwired: 10 in]
        n153 = call <vilib>:"Digital Write Pin.vi"("Arduino Resource"=w642, "Digital I/O Pin (0)"=u8 12, "Value (0)"=u8 0, "error in"=w641) -> ("Arduino Resource"=w658:T1, "error out"=w657:errorcluster)  [unwired: 10 in]
        n154 = call <vilib>:"Digital Write Pin.vi"("Arduino Resource"=w658, "Digital I/O Pin (0)"=u8 12, "Value (0)"=u8 1, "error in"=w657) -> ("Arduino Resource"=w652:T1, "error out"=w651:errorcluster)  [unwired: 10 in]
      }
      frame 26 {
        n155 = call <vilib>:"Digital Write Pin.vi"("Arduino Resource"=w666, "Digital I/O Pin (0)"=u8 2, "Value (0)"=u8 1, "error in"=w665) -> ("Arduino Resource"=w668:T1, "error out"=w667:errorcluster)  [unwired: 10 in]
        n156 = call <vilib>:"Digital Write Pin.vi"("Arduino Resource"=w668, "Digital I/O Pin (0)"=u8 10, "Value (0)"=u8 0, "error in"=w667) -> ("Arduino Resource"=w676:T1, "error out"=w675:errorcluster)  [unwired: 10 in]
        n157 = call <vilib>:"Digital Write Pin.vi"("Arduino Resource"=w676, "Digital I/O Pin (0)"=u8 11, "Value (0)"=u8 0, "error in"=w675) -> ("Arduino Resource"=w677:T1, "error out"=w678:errorcluster)  [unwired: 10 in]
        n158 = call <vilib>:"Digital Write Pin.vi"("Arduino Resource"=w677, "Digital I/O Pin (0)"=u8 12, "Value (0)"=u8 0, "error in"=w678) -> ("Arduino Resource"=w680:T1, "error out"=w679:errorcluster)  [unwired: 10 in]
        n159 = call <vilib>:"Digital Write Pin.vi"("Arduino Resource"=w680, "Digital I/O Pin (0)"=u8 12, "Value (0)"=u8 1, "error in"=w679) -> ("Arduino Resource"=w664:T1, "error out"=w663:errorcluster)  [unwired: 10 in]
      }
      frame 27 {
        n160 = call <vilib>:"Digital Write Pin.vi"("Arduino Resource"=w692, "Digital I/O Pin (0)"=u8 3, "Value (0)"=u8 1, "error in"=w691) -> ("Arduino Resource"=w693:T1, "error out"=w690:errorcluster)  [unwired: 10 in]
        n161 = call <vilib>:"Digital Write Pin.vi"("Arduino Resource"=w693, "Digital I/O Pin (0)"=u8 10, "Value (0)"=u8 0, "error in"=w690) -> ("Arduino Resource"=w700:T1, "error out"=w689:errorcluster)  [unwired: 10 in]
        n162 = call <vilib>:"Digital Write Pin.vi"("Arduino Resource"=w700, "Digital I/O Pin (0)"=u8 11, "Value (0)"=u8 0, "error in"=w689) -> ("Arduino Resource"=w701:T1, "error out"=w688:errorcluster)  [unwired: 10 in]
        n163 = call <vilib>:"Digital Write Pin.vi"("Arduino Resource"=w701, "Digital I/O Pin (0)"=u8 12, "Value (0)"=u8 0, "error in"=w688) -> ("Arduino Resource"=w702:T1, "error out"=w687:errorcluster)  [unwired: 10 in]
        n164 = call <vilib>:"Digital Write Pin.vi"("Arduino Resource"=w702, "Digital I/O Pin (0)"=u8 12, "Value (0)"=u8 1, "error in"=w687) -> ("Arduino Resource"=w686:T1, "error out"=w685:errorcluster)  [unwired: 10 in]
      }
      frame 28 {
        n165 = call <vilib>:"Digital Write Pin.vi"("Arduino Resource"=w710, "Digital I/O Pin (0)"=u8 4, "Value (0)"=u8 1, "error in"=w709) -> ("Arduino Resource"=w712:T1, "error out"=w711:errorcluster)  [unwired: 10 in]
        n166 = call <vilib>:"Digital Write Pin.vi"("Arduino Resource"=w712, "Digital I/O Pin (0)"=u8 10, "Value (0)"=u8 0, "error in"=w711) -> ("Arduino Resource"=w720:T1, "error out"=w719:errorcluster)  [unwired: 10 in]
        n167 = call <vilib>:"Digital Write Pin.vi"("Arduino Resource"=w720, "Digital I/O Pin (0)"=u8 11, "Value (0)"=u8 0, "error in"=w719) -> ("Arduino Resource"=w721:T1, "error out"=w722:errorcluster)  [unwired: 10 in]
        n168 = call <vilib>:"Digital Write Pin.vi"("Arduino Resource"=w721, "Digital I/O Pin (0)"=u8 12, "Value (0)"=u8 0, "error in"=w722) -> ("Arduino Resource"=w724:T1, "error out"=w723:errorcluster)  [unwired: 10 in]
        n169 = call <vilib>:"Digital Write Pin.vi"("Arduino Resource"=w724, "Digital I/O Pin (0)"=u8 12, "Value (0)"=u8 1, "error in"=w723) -> ("Arduino Resource"=w708:T1, "error out"=w707:errorcluster)  [unwired: 10 in]
      }
      frame 29 {
        n170 = call <vilib>:"Digital Write Pin.vi"("Arduino Resource"=w732, "Digital I/O Pin (0)"=u8 5, "Value (0)"=u8 1, "error in"=w731) -> ("Arduino Resource"=w734:T1, "error out"=w733:errorcluster)  [unwired: 10 in]
        n171 = call <vilib>:"Digital Write Pin.vi"("Arduino Resource"=w734, "Digital I/O Pin (0)"=u8 10, "Value (0)"=u8 0, "error in"=w733) -> ("Arduino Resource"=w742:T1, "error out"=w741:errorcluster)  [unwired: 10 in]
        n172 = call <vilib>:"Digital Write Pin.vi"("Arduino Resource"=w742, "Digital I/O Pin (0)"=u8 11, "Value (0)"=u8 0, "error in"=w741) -> ("Arduino Resource"=w743:T1, "error out"=w744:errorcluster)  [unwired: 10 in]
        n173 = call <vilib>:"Digital Write Pin.vi"("Arduino Resource"=w743, "Digital I/O Pin (0)"=u8 12, "Value (0)"=u8 0, "error in"=w744) -> ("Arduino Resource"=w746:T1, "error out"=w745:errorcluster)  [unwired: 10 in]
        n174 = call <vilib>:"Digital Write Pin.vi"("Arduino Resource"=w746, "Digital I/O Pin (0)"=u8 12, "Value (0)"=u8 1, "error in"=w745) -> ("Arduino Resource"=w730:T1, "error out"=w729:errorcluster)  [unwired: 10 in]
      }
      frame 30 {
        n175 = call <vilib>:"Digital Write Pin.vi"("Arduino Resource"=w754, "Digital I/O Pin (0)"=u8 6, "Value (0)"=u8 1, "error in"=w753) -> ("Arduino Resource"=w771:T1, "error out"=w772:errorcluster)  [unwired: 10 in]
        n176 = call <vilib>:"Digital Write Pin.vi"("Arduino Resource"=w771, "Digital I/O Pin (0)"=u8 10, "Value (0)"=u8 0, "error in"=w772) -> ("Arduino Resource"=w769:T1, "error out"=w770:errorcluster)  [unwired: 10 in]
        n177 = call <vilib>:"Digital Write Pin.vi"("Arduino Resource"=w769, "Digital I/O Pin (0)"=u8 11, "Value (0)"=u8 0, "error in"=w770) -> ("Arduino Resource"=w768:T1, "error out"=w767:errorcluster)  [unwired: 10 in]
        n178 = call <vilib>:"Digital Write Pin.vi"("Arduino Resource"=w768, "Digital I/O Pin (0)"=u8 12, "Value (0)"=u8 0, "error in"=w767) -> ("Arduino Resource"=w765:T1, "error out"=w766:errorcluster)  [unwired: 10 in]
        n179 = call <vilib>:"Digital Write Pin.vi"("Arduino Resource"=w765, "Digital I/O Pin (0)"=u8 12, "Value (0)"=u8 1, "error in"=w766) -> ("Arduino Resource"=w751:T1, "error out"=w752:errorcluster)  [unwired: 10 in]
      }
      frame 31 {
        n180 = call <vilib>:"Digital Write Pin.vi"("Arduino Resource"=w776, "Digital I/O Pin (0)"=u8 7, "Value (0)"=u8 1, "error in"=w775) -> ("Arduino Resource"=w778:T1, "error out"=w777:errorcluster)  [unwired: 10 in]
        n181 = call <vilib>:"Digital Write Pin.vi"("Arduino Resource"=w778, "Digital I/O Pin (0)"=u8 10, "Value (0)"=u8 0, "error in"=w777) -> ("Arduino Resource"=w786:T1, "error out"=w785:errorcluster)  [unwired: 10 in]
        n182 = call <vilib>:"Digital Write Pin.vi"("Arduino Resource"=w786, "Digital I/O Pin (0)"=u8 11, "Value (0)"=u8 0, "error in"=w785) -> ("Arduino Resource"=w787:T1, "error out"=w788:errorcluster)  [unwired: 10 in]
        n183 = call <vilib>:"Digital Write Pin.vi"("Arduino Resource"=w787, "Digital I/O Pin (0)"=u8 12, "Value (0)"=u8 0, "error in"=w788) -> ("Arduino Resource"=w790:T1, "error out"=w789:errorcluster)  [unwired: 10 in]
        n184 = call <vilib>:"Digital Write Pin.vi"("Arduino Resource"=w790, "Digital I/O Pin (0)"=u8 12, "Value (0)"=u8 1, "error in"=w789) -> ("Arduino Resource"=w774:T1, "error out"=w773:errorcluster)  [unwired: 10 in]
      }
      frame 32 {
        n185 = call <vilib>:"Digital Write Pin.vi"("Arduino Resource"=w798, "Digital I/O Pin (0)"=u8 8, "Value (0)"=u8 1, "error in"=w797) -> ("Arduino Resource"=w800:T1, "error out"=w799:errorcluster)  [unwired: 10 in]
        n186 = call <vilib>:"Digital Write Pin.vi"("Arduino Resource"=w800, "Digital I/O Pin (0)"=u8 10, "Value (0)"=u8 0, "error in"=w799) -> ("Arduino Resource"=w808:T1, "error out"=w807:errorcluster)  [unwired: 10 in]
        n187 = call <vilib>:"Digital Write Pin.vi"("Arduino Resource"=w808, "Digital I/O Pin (0)"=u8 11, "Value (0)"=u8 0, "error in"=w807) -> ("Arduino Resource"=w809:T1, "error out"=w810:errorcluster)  [unwired: 10 in]
        n188 = call <vilib>:"Digital Write Pin.vi"("Arduino Resource"=w809, "Digital I/O Pin (0)"=u8 12, "Value (0)"=u8 0, "error in"=w810) -> ("Arduino Resource"=w812:T1, "error out"=w811:errorcluster)  [unwired: 10 in]
        n189 = call <vilib>:"Digital Write Pin.vi"("Arduino Resource"=w812, "Digital I/O Pin (0)"=u8 12, "Value (0)"=u8 1, "error in"=w811) -> ("Arduino Resource"=w796:T1, "error out"=w795:errorcluster)  [unwired: 10 in]
      }
      frame 33 {
        n190 = call <vilib>:"Digital Write Pin.vi"("Arduino Resource"=w820, "Digital I/O Pin (0)"=u8 9, "Value (0)"=u8 1, "error in"=w819) -> ("Arduino Resource"=w854:T1, "error out"=w853:errorcluster)  [unwired: 10 in]
        n191 = call <vilib>:"Digital Write Pin.vi"("Arduino Resource"=w854, "Digital I/O Pin (0)"=u8 10, "Value (0)"=u8 0, "error in"=w853) -> ("Arduino Resource"=w862:T1, "error out"=w861:errorcluster)  [unwired: 10 in]
        n192 = call <vilib>:"Digital Write Pin.vi"("Arduino Resource"=w862, "Digital I/O Pin (0)"=u8 11, "Value (0)"=u8 0, "error in"=w861) -> ("Arduino Resource"=w863:T1, "error out"=w864:errorcluster)  [unwired: 10 in]
        n193 = call <vilib>:"Digital Write Pin.vi"("Arduino Resource"=w863, "Digital I/O Pin (0)"=u8 12, "Value (0)"=u8 0, "error in"=w864) -> ("Arduino Resource"=w866:T1, "error out"=w865:errorcluster)  [unwired: 10 in]
        n194 = call <vilib>:"Digital Write Pin.vi"("Arduino Resource"=w866, "Digital I/O Pin (0)"=u8 12, "Value (0)"=u8 1, "error in"=w865) -> ("Arduino Resource"=w822:T1, "error out"=w821:errorcluster)  [unwired: 10 in]
        n195 = call <vilib>:"Digital Write Pin.vi"("Arduino Resource"=w822, "Digital I/O Pin (0)"=u8 2, "Value (0)"=u8 0, "error in"=w821) -> ("Arduino Resource"=w852:T1, "error out"=w851:errorcluster)  [unwired: 10 in]
        n196 = call <vilib>:"Digital Write Pin.vi"("Arduino Resource"=w852, "Digital I/O Pin (0)"=u8 3, "Value (0)"=u8 0, "error in"=w851) -> ("Arduino Resource"=w850:T1, "error out"=w849:errorcluster)  [unwired: 10 in]
        n197 = call <vilib>:"Digital Write Pin.vi"("Arduino Resource"=w850, "Digital I/O Pin (0)"=u8 4, "Value (0)"=u8 0, "error in"=w849) -> ("Arduino Resource"=w848:T1, "error out"=w847:errorcluster)  [unwired: 10 in]
        n198 = call <vilib>:"Digital Write Pin.vi"("Arduino Resource"=w848, "Digital I/O Pin (0)"=u8 5, "Value (0)"=u8 0, "error in"=w847) -> ("Arduino Resource"=w846:T1, "error out"=w845:errorcluster)  [unwired: 10 in]
        n199 = call <vilib>:"Digital Write Pin.vi"("Arduino Resource"=w846, "Digital I/O Pin (0)"=u8 6, "Value (0)"=u8 0, "error in"=w845) -> ("Arduino Resource"=w844:T1, "error out"=w843:errorcluster)  [unwired: 10 in]
        n200 = call <vilib>:"Digital Write Pin.vi"("Arduino Resource"=w844, "Digital I/O Pin (0)"=u8 7, "Value (0)"=u8 0, "error in"=w843) -> ("Arduino Resource"=w842:T1, "error out"=w841:errorcluster)  [unwired: 10 in]
        n201 = call <vilib>:"Digital Write Pin.vi"("Arduino Resource"=w842, "Digital I/O Pin (0)"=u8 8, "Value (0)"=u8 0, "error in"=w841) -> ("Arduino Resource"=w840:T1, "error out"=w839:errorcluster)  [unwired: 10 in]
        n202 = call <vilib>:"Digital Write Pin.vi"("Arduino Resource"=w840, "Digital I/O Pin (0)"=u8 9, "Value (0)"=u8 0, "error in"=w839) -> ("Arduino Resource"=w818:T1, "error out"=w817:errorcluster)  [unwired: 10 in]
      }
      frame 34 {
        n203 = call <vilib>:"Digital Write Pin.vi"("Arduino Resource"=w874, "Digital I/O Pin (0)"=u8 2, "Value (0)"=u8 1, "error in"=w873) -> ("Arduino Resource"=w876:T1, "error out"=w875:errorcluster)  [unwired: 10 in]
        n204 = call <vilib>:"Digital Write Pin.vi"("Arduino Resource"=w876, "Digital I/O Pin (0)"=u8 10, "Value (0)"=u8 0, "error in"=w875) -> ("Arduino Resource"=w884:T1, "error out"=w883:errorcluster)  [unwired: 10 in]
        n205 = call <vilib>:"Digital Write Pin.vi"("Arduino Resource"=w884, "Digital I/O Pin (0)"=u8 11, "Value (0)"=u8 1, "error in"=w883) -> ("Arduino Resource"=w885:T1, "error out"=w886:errorcluster)  [unwired: 10 in]
        n206 = call <vilib>:"Digital Write Pin.vi"("Arduino Resource"=w885, "Digital I/O Pin (0)"=u8 12, "Value (0)"=u8 0, "error in"=w886) -> ("Arduino Resource"=w888:T1, "error out"=w887:errorcluster)  [unwired: 10 in]
        n207 = call <vilib>:"Digital Write Pin.vi"("Arduino Resource"=w888, "Digital I/O Pin (0)"=u8 12, "Value (0)"=u8 1, "error in"=w887) -> ("Arduino Resource"=w872:T1, "error out"=w871:errorcluster)  [unwired: 10 in]
      }
      frame 35 {
        n208 = call <vilib>:"Digital Write Pin.vi"("Arduino Resource"=w896, "Digital I/O Pin (0)"=u8 3, "Value (0)"=u8 1, "error in"=w895) -> ("Arduino Resource"=w898:T1, "error out"=w897:errorcluster)  [unwired: 10 in]
        n209 = call <vilib>:"Digital Write Pin.vi"("Arduino Resource"=w898, "Digital I/O Pin (0)"=u8 10, "Value (0)"=u8 0, "error in"=w897) -> ("Arduino Resource"=w906:T1, "error out"=w905:errorcluster)  [unwired: 10 in]
        n210 = call <vilib>:"Digital Write Pin.vi"("Arduino Resource"=w906, "Digital I/O Pin (0)"=u8 11, "Value (0)"=u8 1, "error in"=w905) -> ("Arduino Resource"=w907:T1, "error out"=w908:errorcluster)  [unwired: 10 in]
        n211 = call <vilib>:"Digital Write Pin.vi"("Arduino Resource"=w907, "Digital I/O Pin (0)"=u8 12, "Value (0)"=u8 0, "error in"=w908) -> ("Arduino Resource"=w910:T1, "error out"=w909:errorcluster)  [unwired: 10 in]
        n212 = call <vilib>:"Digital Write Pin.vi"("Arduino Resource"=w910, "Digital I/O Pin (0)"=u8 12, "Value (0)"=u8 1, "error in"=w909) -> ("Arduino Resource"=w894:T1, "error out"=w893:errorcluster)  [unwired: 10 in]
      }
      frame 36 {
        n213 = call <vilib>:"Digital Write Pin.vi"("Arduino Resource"=w918, "Digital I/O Pin (0)"=u8 4, "Value (0)"=u8 1, "error in"=w917) -> ("Arduino Resource"=w920:T1, "error out"=w919:errorcluster)  [unwired: 10 in]
        n214 = call <vilib>:"Digital Write Pin.vi"("Arduino Resource"=w920, "Digital I/O Pin (0)"=u8 10, "Value (0)"=u8 0, "error in"=w919) -> ("Arduino Resource"=w928:T1, "error out"=w927:errorcluster)  [unwired: 10 in]
        n215 = call <vilib>:"Digital Write Pin.vi"("Arduino Resource"=w928, "Digital I/O Pin (0)"=u8 11, "Value (0)"=u8 1, "error in"=w927) -> ("Arduino Resource"=w929:T1, "error out"=w930:errorcluster)  [unwired: 10 in]
        n216 = call <vilib>:"Digital Write Pin.vi"("Arduino Resource"=w929, "Digital I/O Pin (0)"=u8 12, "Value (0)"=u8 0, "error in"=w930) -> ("Arduino Resource"=w932:T1, "error out"=w931:errorcluster)  [unwired: 10 in]
        n217 = call <vilib>:"Digital Write Pin.vi"("Arduino Resource"=w932, "Digital I/O Pin (0)"=u8 12, "Value (0)"=u8 1, "error in"=w931) -> ("Arduino Resource"=w916:T1, "error out"=w915:errorcluster)  [unwired: 10 in]
      }
      frame 37 {
        n218 = call <vilib>:"Digital Write Pin.vi"("Arduino Resource"=w940, "Digital I/O Pin (0)"=u8 5, "Value (0)"=u8 1, "error in"=w939) -> ("Arduino Resource"=w942:T1, "error out"=w941:errorcluster)  [unwired: 10 in]
        n219 = call <vilib>:"Digital Write Pin.vi"("Arduino Resource"=w942, "Digital I/O Pin (0)"=u8 10, "Value (0)"=u8 0, "error in"=w941) -> ("Arduino Resource"=w950:T1, "error out"=w949:errorcluster)  [unwired: 10 in]
        n220 = call <vilib>:"Digital Write Pin.vi"("Arduino Resource"=w950, "Digital I/O Pin (0)"=u8 11, "Value (0)"=u8 1, "error in"=w949) -> ("Arduino Resource"=w951:T1, "error out"=w952:errorcluster)  [unwired: 10 in]
        n221 = call <vilib>:"Digital Write Pin.vi"("Arduino Resource"=w951, "Digital I/O Pin (0)"=u8 12, "Value (0)"=u8 0, "error in"=w952) -> ("Arduino Resource"=w954:T1, "error out"=w953:errorcluster)  [unwired: 10 in]
        n222 = call <vilib>:"Digital Write Pin.vi"("Arduino Resource"=w954, "Digital I/O Pin (0)"=u8 12, "Value (0)"=u8 1, "error in"=w953) -> ("Arduino Resource"=w938:T1, "error out"=w937:errorcluster)  [unwired: 10 in]
      }
      frame 38 {
        n223 = call <vilib>:"Digital Write Pin.vi"("Arduino Resource"=w962, "Digital I/O Pin (0)"=u8 9, "Value (0)"=u8 1, "error in"=w961) -> ("Arduino Resource"=w964:T1, "error out"=w963:errorcluster)  [unwired: 10 in]
        n224 = call <vilib>:"Digital Write Pin.vi"("Arduino Resource"=w964, "Digital I/O Pin (0)"=u8 10, "Value (0)"=u8 0, "error in"=w963) -> ("Arduino Resource"=w972:T1, "error out"=w971:errorcluster)  [unwired: 10 in]
        n225 = call <vilib>:"Digital Write Pin.vi"("Arduino Resource"=w972, "Digital I/O Pin (0)"=u8 11, "Value (0)"=u8 1, "error in"=w971) -> ("Arduino Resource"=w973:T1, "error out"=w974:errorcluster)  [unwired: 10 in]
        n226 = call <vilib>:"Digital Write Pin.vi"("Arduino Resource"=w973, "Digital I/O Pin (0)"=u8 12, "Value (0)"=u8 0, "error in"=w974) -> ("Arduino Resource"=w976:T1, "error out"=w975:errorcluster)  [unwired: 10 in]
        n227 = call <vilib>:"Digital Write Pin.vi"("Arduino Resource"=w976, "Digital I/O Pin (0)"=u8 12, "Value (0)"=u8 1, "error in"=w975) -> ("Arduino Resource"=w960:T1, "error out"=w959:errorcluster)  [unwired: 10 in]
      }
      frame 39 {
        n228 = call <vilib>:"Digital Write Pin.vi"("Arduino Resource"=w984, "Digital I/O Pin (0)"=u8 8, "Value (0)"=u8 1, "error in"=w983) -> ("Arduino Resource"=w986:T1, "error out"=w985:errorcluster)  [unwired: 10 in]
        n229 = call <vilib>:"Digital Write Pin.vi"("Arduino Resource"=w986, "Digital I/O Pin (0)"=u8 10, "Value (0)"=u8 0, "error in"=w985) -> ("Arduino Resource"=w994:T1, "error out"=w993:errorcluster)  [unwired: 10 in]
        n230 = call <vilib>:"Digital Write Pin.vi"("Arduino Resource"=w994, "Digital I/O Pin (0)"=u8 11, "Value (0)"=u8 1, "error in"=w993) -> ("Arduino Resource"=w995:T1, "error out"=w996:errorcluster)  [unwired: 10 in]
        n231 = call <vilib>:"Digital Write Pin.vi"("Arduino Resource"=w995, "Digital I/O Pin (0)"=u8 12, "Value (0)"=u8 0, "error in"=w996) -> ("Arduino Resource"=w998:T1, "error out"=w997:errorcluster)  [unwired: 10 in]
        n232 = call <vilib>:"Digital Write Pin.vi"("Arduino Resource"=w998, "Digital I/O Pin (0)"=u8 12, "Value (0)"=u8 1, "error in"=w997) -> ("Arduino Resource"=w982:T1, "error out"=w981:errorcluster)  [unwired: 10 in]
      }
      frame 40 {
        n233 = call <vilib>:"Digital Write Pin.vi"("Arduino Resource"=w1006, "Digital I/O Pin (0)"=u8 7, "Value (0)"=u8 1, "error in"=w1005) -> ("Arduino Resource"=w1008:T1, "error out"=w1007:errorcluster)  [unwired: 10 in]
        n234 = call <vilib>:"Digital Write Pin.vi"("Arduino Resource"=w1008, "Digital I/O Pin (0)"=u8 10, "Value (0)"=u8 0, "error in"=w1007) -> ("Arduino Resource"=w1016:T1, "error out"=w1015:errorcluster)  [unwired: 10 in]
        n235 = call <vilib>:"Digital Write Pin.vi"("Arduino Resource"=w1016, "Digital I/O Pin (0)"=u8 11, "Value (0)"=u8 1, "error in"=w1015) -> ("Arduino Resource"=w1017:T1, "error out"=w1018:errorcluster)  [unwired: 10 in]
        n236 = call <vilib>:"Digital Write Pin.vi"("Arduino Resource"=w1017, "Digital I/O Pin (0)"=u8 12, "Value (0)"=u8 0, "error in"=w1018) -> ("Arduino Resource"=w1020:T1, "error out"=w1019:errorcluster)  [unwired: 10 in]
        n237 = call <vilib>:"Digital Write Pin.vi"("Arduino Resource"=w1020, "Digital I/O Pin (0)"=u8 12, "Value (0)"=u8 1, "error in"=w1019) -> ("Arduino Resource"=w1004:T1, "error out"=w1003:errorcluster)  [unwired: 10 in]
      }
      frame 41 {
        n238 = call <vilib>:"Digital Write Pin.vi"("Arduino Resource"=w1028, "Digital I/O Pin (0)"=u8 6, "Value (0)"=u8 1, "error in"=w1027) -> ("Arduino Resource"=w1064:T1, "error out"=w1063:errorcluster)  [unwired: 10 in]
        n239 = call <vilib>:"Digital Write Pin.vi"("Arduino Resource"=w1064, "Digital I/O Pin (0)"=u8 10, "Value (0)"=u8 0, "error in"=w1063) -> ("Arduino Resource"=w1070:T1, "error out"=w1069:errorcluster)  [unwired: 10 in]
        n240 = call <vilib>:"Digital Write Pin.vi"("Arduino Resource"=w1070, "Digital I/O Pin (0)"=u8 11, "Value (0)"=u8 1, "error in"=w1069) -> ("Arduino Resource"=w1062:T1, "error out"=w1061:errorcluster)  [unwired: 10 in]
        n241 = call <vilib>:"Digital Write Pin.vi"("Arduino Resource"=w1062, "Digital I/O Pin (0)"=u8 12, "Value (0)"=u8 0, "error in"=w1061) -> ("Arduino Resource"=w1074:T1, "error out"=w1073:errorcluster)  [unwired: 10 in]
        n242 = call <vilib>:"Digital Write Pin.vi"("Arduino Resource"=w1074, "Digital I/O Pin (0)"=u8 12, "Value (0)"=u8 1, "error in"=w1073) -> ("Arduino Resource"=w1030:T1, "error out"=w1029:errorcluster)  [unwired: 10 in]
        n243 = call <vilib>:"Digital Write Pin.vi"("Arduino Resource"=w1030, "Digital I/O Pin (0)"=u8 2, "Value (0)"=u8 0, "error in"=w1029) -> ("Arduino Resource"=w1060:T1, "error out"=w1059:errorcluster)  [unwired: 10 in]
        n244 = call <vilib>:"Digital Write Pin.vi"("Arduino Resource"=w1060, "Digital I/O Pin (0)"=u8 3, "Value (0)"=u8 0, "error in"=w1059) -> ("Arduino Resource"=w1058:T1, "error out"=w1057:errorcluster)  [unwired: 10 in]
        n245 = call <vilib>:"Digital Write Pin.vi"("Arduino Resource"=w1058, "Digital I/O Pin (0)"=u8 4, "Value (0)"=u8 0, "error in"=w1057) -> ("Arduino Resource"=w1056:T1, "error out"=w1055:errorcluster)  [unwired: 10 in]
        n246 = call <vilib>:"Digital Write Pin.vi"("Arduino Resource"=w1056, "Digital I/O Pin (0)"=u8 5, "Value (0)"=u8 0, "error in"=w1055) -> ("Arduino Resource"=w1054:T1, "error out"=w1053:errorcluster)  [unwired: 10 in]
        n247 = call <vilib>:"Digital Write Pin.vi"("Arduino Resource"=w1054, "Digital I/O Pin (0)"=u8 6, "Value (0)"=u8 0, "error in"=w1053) -> ("Arduino Resource"=w1052:T1, "error out"=w1051:errorcluster)  [unwired: 10 in]
        n248 = call <vilib>:"Digital Write Pin.vi"("Arduino Resource"=w1052, "Digital I/O Pin (0)"=u8 7, "Value (0)"=u8 0, "error in"=w1051) -> ("Arduino Resource"=w1050:T1, "error out"=w1049:errorcluster)  [unwired: 10 in]
        n249 = call <vilib>:"Digital Write Pin.vi"("Arduino Resource"=w1050, "Digital I/O Pin (0)"=u8 8, "Value (0)"=u8 0, "error in"=w1049) -> ("Arduino Resource"=w1048:T1, "error out"=w1047:errorcluster)  [unwired: 10 in]
        n250 = call <vilib>:"Digital Write Pin.vi"("Arduino Resource"=w1048, "Digital I/O Pin (0)"=u8 9, "Value (0)"=u8 0, "error in"=w1047) -> ("Arduino Resource"=w1026:T1, "error out"=w1025:errorcluster)  [unwired: 10 in]
      }
      frame 42 {
        n251 = call <vilib>:"Digital Write Pin.vi"("Arduino Resource"=w1086, "Digital I/O Pin (0)"=u8 9, "Value (0)"=u8 1, "error in"=w1085) -> ("Arduino Resource"=w1089:T1, "error out"=w1084:errorcluster)  [unwired: 10 in]
        n252 = call <vilib>:"Digital Write Pin.vi"("Arduino Resource"=w1089, "Digital I/O Pin (0)"=u8 10, "Value (0)"=u8 1, "error in"=w1084) -> ("Arduino Resource"=w1088:T1, "error out"=w1083:errorcluster)  [unwired: 10 in]
        n253 = call <vilib>:"Digital Write Pin.vi"("Arduino Resource"=w1088, "Digital I/O Pin (0)"=u8 11, "Value (0)"=u8 0, "error in"=w1083) -> ("Arduino Resource"=w1087:T1, "error out"=w1082:errorcluster)  [unwired: 10 in]
        n254 = call <vilib>:"Digital Write Pin.vi"("Arduino Resource"=w1087, "Digital I/O Pin (0)"=u8 12, "Value (0)"=u8 0, "error in"=w1082) -> ("Arduino Resource"=w1096:T1, "error out"=w1081:errorcluster)  [unwired: 10 in]
        n255 = call <vilib>:"Digital Write Pin.vi"("Arduino Resource"=w1096, "Digital I/O Pin (0)"=u8 12, "Value (0)"=u8 1, "error in"=w1081) -> ("Arduino Resource"=w1080:T1, "error out"=w1079:errorcluster)  [unwired: 10 in]
      }
      frame 43 {
        n256 = call <vilib>:"Digital Write Pin.vi"("Arduino Resource"=w1104, "Digital I/O Pin (0)"=u8 8, "Value (0)"=u8 1, "error in"=w1103) -> ("Arduino Resource"=w1108:T1, "error out"=w1107:errorcluster)  [unwired: 10 in]
        n257 = call <vilib>:"Digital Write Pin.vi"("Arduino Resource"=w1108, "Digital I/O Pin (0)"=u8 10, "Value (0)"=u8 1, "error in"=w1107) -> ("Arduino Resource"=w1109:T1, "error out"=w1114:errorcluster)  [unwired: 10 in]
        n258 = call <vilib>:"Digital Write Pin.vi"("Arduino Resource"=w1109, "Digital I/O Pin (0)"=u8 11, "Value (0)"=u8 0, "error in"=w1114) -> ("Arduino Resource"=w1106:T1, "error out"=w1105:errorcluster)  [unwired: 10 in]
        n259 = call <vilib>:"Digital Write Pin.vi"("Arduino Resource"=w1106, "Digital I/O Pin (0)"=u8 12, "Value (0)"=u8 0, "error in"=w1105) -> ("Arduino Resource"=w1118:T1, "error out"=w1117:errorcluster)  [unwired: 10 in]
        n260 = call <vilib>:"Digital Write Pin.vi"("Arduino Resource"=w1118, "Digital I/O Pin (0)"=u8 12, "Value (0)"=u8 1, "error in"=w1117) -> ("Arduino Resource"=w1102:T1, "error out"=w1101:errorcluster)  [unwired: 10 in]
      }
      frame 44 {
        n261 = call <vilib>:"Digital Write Pin.vi"("Arduino Resource"=w1126, "Digital I/O Pin (0)"=u8 7, "Value (0)"=u8 1, "error in"=w1125) -> ("Arduino Resource"=w1130:T1, "error out"=w1129:errorcluster)  [unwired: 10 in]
        n262 = call <vilib>:"Digital Write Pin.vi"("Arduino Resource"=w1130, "Digital I/O Pin (0)"=u8 10, "Value (0)"=u8 1, "error in"=w1129) -> ("Arduino Resource"=w1131:T1, "error out"=w1136:errorcluster)  [unwired: 10 in]
        n263 = call <vilib>:"Digital Write Pin.vi"("Arduino Resource"=w1131, "Digital I/O Pin (0)"=u8 11, "Value (0)"=u8 0, "error in"=w1136) -> ("Arduino Resource"=w1128:T1, "error out"=w1127:errorcluster)  [unwired: 10 in]
        n264 = call <vilib>:"Digital Write Pin.vi"("Arduino Resource"=w1128, "Digital I/O Pin (0)"=u8 12, "Value (0)"=u8 0, "error in"=w1127) -> ("Arduino Resource"=w1140:T1, "error out"=w1139:errorcluster)  [unwired: 10 in]
        n265 = call <vilib>:"Digital Write Pin.vi"("Arduino Resource"=w1140, "Digital I/O Pin (0)"=u8 12, "Value (0)"=u8 1, "error in"=w1139) -> ("Arduino Resource"=w1124:T1, "error out"=w1123:errorcluster)  [unwired: 10 in]
      }
      frame 45 {
        n266 = call <vilib>:"Digital Write Pin.vi"("Arduino Resource"=w1148, "Digital I/O Pin (0)"=u8 6, "Value (0)"=u8 1, "error in"=w1147) -> ("Arduino Resource"=w1152:T1, "error out"=w1151:errorcluster)  [unwired: 10 in]
        n267 = call <vilib>:"Digital Write Pin.vi"("Arduino Resource"=w1152, "Digital I/O Pin (0)"=u8 10, "Value (0)"=u8 1, "error in"=w1151) -> ("Arduino Resource"=w1153:T1, "error out"=w1158:errorcluster)  [unwired: 10 in]
        n268 = call <vilib>:"Digital Write Pin.vi"("Arduino Resource"=w1153, "Digital I/O Pin (0)"=u8 11, "Value (0)"=u8 0, "error in"=w1158) -> ("Arduino Resource"=w1150:T1, "error out"=w1149:errorcluster)  [unwired: 10 in]
        n269 = call <vilib>:"Digital Write Pin.vi"("Arduino Resource"=w1150, "Digital I/O Pin (0)"=u8 12, "Value (0)"=u8 0, "error in"=w1149) -> ("Arduino Resource"=w1162:T1, "error out"=w1161:errorcluster)  [unwired: 10 in]
        n270 = call <vilib>:"Digital Write Pin.vi"("Arduino Resource"=w1162, "Digital I/O Pin (0)"=u8 12, "Value (0)"=u8 1, "error in"=w1161) -> ("Arduino Resource"=w1146:T1, "error out"=w1145:errorcluster)  [unwired: 10 in]
      }
      frame 46 {
        n271 = call <vilib>:"Digital Write Pin.vi"("Arduino Resource"=w1170, "Digital I/O Pin (0)"=u8 5, "Value (0)"=u8 1, "error in"=w1169) -> ("Arduino Resource"=w1174:T1, "error out"=w1173:errorcluster)  [unwired: 10 in]
        n272 = call <vilib>:"Digital Write Pin.vi"("Arduino Resource"=w1174, "Digital I/O Pin (0)"=u8 10, "Value (0)"=u8 1, "error in"=w1173) -> ("Arduino Resource"=w1175:T1, "error out"=w1180:errorcluster)  [unwired: 10 in]
        n273 = call <vilib>:"Digital Write Pin.vi"("Arduino Resource"=w1175, "Digital I/O Pin (0)"=u8 11, "Value (0)"=u8 0, "error in"=w1180) -> ("Arduino Resource"=w1172:T1, "error out"=w1171:errorcluster)  [unwired: 10 in]
        n274 = call <vilib>:"Digital Write Pin.vi"("Arduino Resource"=w1172, "Digital I/O Pin (0)"=u8 12, "Value (0)"=u8 0, "error in"=w1171) -> ("Arduino Resource"=w1184:T1, "error out"=w1183:errorcluster)  [unwired: 10 in]
        n275 = call <vilib>:"Digital Write Pin.vi"("Arduino Resource"=w1184, "Digital I/O Pin (0)"=u8 12, "Value (0)"=u8 1, "error in"=w1183) -> ("Arduino Resource"=w1168:T1, "error out"=w1167:errorcluster)  [unwired: 10 in]
      }
      frame 47 {
        n276 = call <vilib>:"Digital Write Pin.vi"("Arduino Resource"=w1192, "Digital I/O Pin (0)"=u8 4, "Value (0)"=u8 1, "error in"=w1191) -> ("Arduino Resource"=w1196:T1, "error out"=w1195:errorcluster)  [unwired: 10 in]
        n277 = call <vilib>:"Digital Write Pin.vi"("Arduino Resource"=w1196, "Digital I/O Pin (0)"=u8 10, "Value (0)"=u8 1, "error in"=w1195) -> ("Arduino Resource"=w1197:T1, "error out"=w1202:errorcluster)  [unwired: 10 in]
        n278 = call <vilib>:"Digital Write Pin.vi"("Arduino Resource"=w1197, "Digital I/O Pin (0)"=u8 11, "Value (0)"=u8 0, "error in"=w1202) -> ("Arduino Resource"=w1194:T1, "error out"=w1193:errorcluster)  [unwired: 10 in]
        n279 = call <vilib>:"Digital Write Pin.vi"("Arduino Resource"=w1194, "Digital I/O Pin (0)"=u8 12, "Value (0)"=u8 0, "error in"=w1193) -> ("Arduino Resource"=w1206:T1, "error out"=w1205:errorcluster)  [unwired: 10 in]
        n280 = call <vilib>:"Digital Write Pin.vi"("Arduino Resource"=w1206, "Digital I/O Pin (0)"=u8 12, "Value (0)"=u8 1, "error in"=w1205) -> ("Arduino Resource"=w1190:T1, "error out"=w1189:errorcluster)  [unwired: 10 in]
      }
      frame 48 {
        n281 = call <vilib>:"Digital Write Pin.vi"("Arduino Resource"=w1214, "Digital I/O Pin (0)"=u8 3, "Value (0)"=u8 1, "error in"=w1213) -> ("Arduino Resource"=w1229:T1, "error out"=w1230:errorcluster)  [unwired: 10 in]
        n282 = call <vilib>:"Digital Write Pin.vi"("Arduino Resource"=w1229, "Digital I/O Pin (0)"=u8 10, "Value (0)"=u8 1, "error in"=w1230) -> ("Arduino Resource"=w1228:T1, "error out"=w1227:errorcluster)  [unwired: 10 in]
        n283 = call <vilib>:"Digital Write Pin.vi"("Arduino Resource"=w1228, "Digital I/O Pin (0)"=u8 11, "Value (0)"=u8 0, "error in"=w1227) -> ("Arduino Resource"=w1231:T1, "error out"=w1232:errorcluster)  [unwired: 10 in]
        n284 = call <vilib>:"Digital Write Pin.vi"("Arduino Resource"=w1231, "Digital I/O Pin (0)"=u8 12, "Value (0)"=u8 0, "error in"=w1232) -> ("Arduino Resource"=w1225:T1, "error out"=w1226:errorcluster)  [unwired: 10 in]
        n285 = call <vilib>:"Digital Write Pin.vi"("Arduino Resource"=w1225, "Digital I/O Pin (0)"=u8 12, "Value (0)"=u8 1, "error in"=w1226) -> ("Arduino Resource"=w1212:T1, "error out"=w1211:errorcluster)  [unwired: 10 in]
      }
      frame 49 {
        n286 = call <vilib>:"Digital Write Pin.vi"("Arduino Resource"=w1236, "Digital I/O Pin (0)"=u8 2, "Value (0)"=u8 1, "error in"=w1235) -> ("Arduino Resource"=w1240:T1, "error out"=w1239:errorcluster)  [unwired: 10 in]
        n287 = call <vilib>:"Digital Write Pin.vi"("Arduino Resource"=w1240, "Digital I/O Pin (0)"=u8 10, "Value (0)"=u8 1, "error in"=w1239) -> ("Arduino Resource"=w1241:T1, "error out"=w1246:errorcluster)  [unwired: 10 in]
        n288 = call <vilib>:"Digital Write Pin.vi"("Arduino Resource"=w1241, "Digital I/O Pin (0)"=u8 11, "Value (0)"=u8 0, "error in"=w1246) -> ("Arduino Resource"=w1238:T1, "error out"=w1237:errorcluster)  [unwired: 10 in]
        n289 = call <vilib>:"Digital Write Pin.vi"("Arduino Resource"=w1238, "Digital I/O Pin (0)"=u8 12, "Value (0)"=u8 0, "error in"=w1237) -> ("Arduino Resource"=w1250:T1, "error out"=w1249:errorcluster)  [unwired: 10 in]
        n290 = call <vilib>:"Digital Write Pin.vi"("Arduino Resource"=w1250, "Digital I/O Pin (0)"=u8 12, "Value (0)"=u8 1, "error in"=w1249) -> ("Arduino Resource"=w1234:T1, "error out"=w1233:errorcluster)  [unwired: 10 in]
      }
      frame 2 {
        n291 = call <vilib>:"Digital Write Pin.vi"("Arduino Resource"=w1261, "Digital I/O Pin (0)"=u8 2, "Value (0)"=u8 0, "error in"=w1260) -> ("Arduino Resource"=w1258:T1, "error out"=w1257:errorcluster)  [unwired: 10 in]
        n292 = call <vilib>:"Digital Write Pin.vi"("Arduino Resource"=w1258, "Digital I/O Pin (0)"=u8 10, "Value (0)"=u8 0, "error in"=w1257) -> ("Arduino Resource"=w1268:T1, "error out"=w1267:errorcluster)  [unwired: 10 in]
        n293 = call <vilib>:"Digital Write Pin.vi"("Arduino Resource"=w1268, "Digital I/O Pin (0)"=u8 11, "Value (0)"=u8 0, "error in"=w1267) -> ("Arduino Resource"=w1269:T1, "error out"=w1270:errorcluster)  [unwired: 10 in]
        n294 = call <vilib>:"Digital Write Pin.vi"("Arduino Resource"=w1269, "Digital I/O Pin (0)"=u8 12, "Value (0)"=u8 0, "error in"=w1270) -> ("Arduino Resource"=w1272:T1, "error out"=w1271:errorcluster)  [unwired: 10 in]
        n295 = call <vilib>:"Digital Write Pin.vi"("Arduino Resource"=w1272, "Digital I/O Pin (0)"=u8 12, "Value (0)"=u8 1, "error in"=w1271) -> ("Arduino Resource"=w1256:T1, "error out"=w1255:errorcluster)  [unwired: 10 in]
      }
      frame 1 {
        n296 = call <vilib>:"Digital Write Pin.vi"("Arduino Resource"=w1278, "Digital I/O Pin (0)"=u8 2, "Value (0)"=u8 1, "error in"=w1277) -> ("Arduino Resource"=w1355:T1, "error out"=w1354:errorcluster)  [unwired: 10 in]
        n297 = call <vilib>:"Digital Write Pin.vi"("Arduino Resource"=w1355, "Digital I/O Pin (0)"=u8 3, "Value (0)"=u8 1, "error in"=w1354) -> ("Arduino Resource"=w1353:T1, "error out"=w1352:errorcluster)  [unwired: 10 in]
        n298 = call <vilib>:"Digital Write Pin.vi"("Arduino Resource"=w1353, "Digital I/O Pin (0)"=u8 4, "Value (0)"=u8 1, "error in"=w1352) -> ("Arduino Resource"=w1351:T1, "error out"=w1350:errorcluster)  [unwired: 10 in]
        n299 = call <vilib>:"Digital Write Pin.vi"("Arduino Resource"=w1351, "Digital I/O Pin (0)"=u8 5, "Value (0)"=u8 1, "error in"=w1350) -> ("Arduino Resource"=w1349:T1, "error out"=w1348:errorcluster)  [unwired: 10 in]
        n300 = call <vilib>:"Digital Write Pin.vi"("Arduino Resource"=w1349, "Digital I/O Pin (0)"=u8 6, "Value (0)"=u8 1, "error in"=w1348) -> ("Arduino Resource"=w1347:T1, "error out"=w1346:errorcluster)  [unwired: 10 in]
        n301 = call <vilib>:"Digital Write Pin.vi"("Arduino Resource"=w1347, "Digital I/O Pin (0)"=u8 7, "Value (0)"=u8 1, "error in"=w1346) -> ("Arduino Resource"=w1345:T1, "error out"=w1344:errorcluster)  [unwired: 10 in]
        n302 = call <vilib>:"Digital Write Pin.vi"("Arduino Resource"=w1345, "Digital I/O Pin (0)"=u8 8, "Value (0)"=u8 1, "error in"=w1344) -> ("Arduino Resource"=w1343:T1, "error out"=w1342:errorcluster)  [unwired: 10 in]
        n303 = call <vilib>:"Digital Write Pin.vi"("Arduino Resource"=w1343, "Digital I/O Pin (0)"=u8 9, "Value (0)"=u8 1, "error in"=w1342) -> ("Arduino Resource"=w1341:T1, "error out"=w1340:errorcluster)  [unwired: 10 in]
        n304 = call <vilib>:"Digital Write Pin.vi"("Arduino Resource"=w1341, "Digital I/O Pin (0)"=u8 10, "Value (0)"=u8 0, "error in"=w1340) -> ("Arduino Resource"=w1339:T1, "error out"=w1338:errorcluster)  [unwired: 10 in]
        n305 = call <vilib>:"Digital Write Pin.vi"("Arduino Resource"=w1339, "Digital I/O Pin (0)"=u8 11, "Value (0)"=u8 0, "error in"=w1338) -> ("Arduino Resource"=w1356:T1, "error out"=w1357:errorcluster)  [unwired: 10 in]
        n306 = call <vilib>:"Digital Write Pin.vi"("Arduino Resource"=w1356, "Digital I/O Pin (0)"=u8 12, "Value (0)"=u8 0, "error in"=w1357) -> ("Arduino Resource"=w1359:T1, "error out"=w1358:errorcluster)  [unwired: 10 in]
        n307 = call <vilib>:"Digital Write Pin.vi"("Arduino Resource"=w1359, "Digital I/O Pin (0)"=u8 12, "Value (0)"=u8 1, "error in"=w1358) -> ("Arduino Resource"=w1410:T1, "error out"=w1411:errorcluster)  [unwired: 10 in]
        n308 = call <vilib>:"Digital Write Pin.vi"("Arduino Resource"=w1410, "Digital I/O Pin (0)"=u8 2, "Value (0)"=u8 1, "error in"=w1411) -> ("Arduino Resource"=w1392:T1, "error out"=w1393:errorcluster)  [unwired: 10 in]
        n309 = call <vilib>:"Digital Write Pin.vi"("Arduino Resource"=w1392, "Digital I/O Pin (0)"=u8 3, "Value (0)"=u8 1, "error in"=w1393) -> ("Arduino Resource"=w1391:T1, "error out"=w1394:errorcluster)  [unwired: 10 in]
        n310 = call <vilib>:"Digital Write Pin.vi"("Arduino Resource"=w1391, "Digital I/O Pin (0)"=u8 4, "Value (0)"=u8 1, "error in"=w1394) -> ("Arduino Resource"=w1390:T1, "error out"=w1395:errorcluster)  [unwired: 10 in]
        n311 = call <vilib>:"Digital Write Pin.vi"("Arduino Resource"=w1390, "Digital I/O Pin (0)"=u8 5, "Value (0)"=u8 1, "error in"=w1395) -> ("Arduino Resource"=w1389:T1, "error out"=w1396:errorcluster)  [unwired: 10 in]
        n312 = call <vilib>:"Digital Write Pin.vi"("Arduino Resource"=w1389, "Digital I/O Pin (0)"=u8 6, "Value (0)"=u8 1, "error in"=w1396) -> ("Arduino Resource"=w1388:T1, "error out"=w1397:errorcluster)  [unwired: 10 in]
        n313 = call <vilib>:"Digital Write Pin.vi"("Arduino Resource"=w1388, "Digital I/O Pin (0)"=u8 7, "Value (0)"=u8 1, "error in"=w1397) -> ("Arduino Resource"=w1387:T1, "error out"=w1398:errorcluster)  [unwired: 10 in]
        n314 = call <vilib>:"Digital Write Pin.vi"("Arduino Resource"=w1387, "Digital I/O Pin (0)"=u8 8, "Value (0)"=u8 1, "error in"=w1398) -> ("Arduino Resource"=w1386:T1, "error out"=w1399:errorcluster)  [unwired: 10 in]
        n315 = call <vilib>:"Digital Write Pin.vi"("Arduino Resource"=w1386, "Digital I/O Pin (0)"=u8 9, "Value (0)"=u8 1, "error in"=w1399) -> ("Arduino Resource"=w1385:T1, "error out"=w1400:errorcluster)  [unwired: 10 in]
        n316 = call <vilib>:"Digital Write Pin.vi"("Arduino Resource"=w1385, "Digital I/O Pin (0)"=u8 10, "Value (0)"=u8 0, "error in"=w1400) -> ("Arduino Resource"=w1384:T1, "error out"=w1401:errorcluster)  [unwired: 10 in]
        n317 = call <vilib>:"Digital Write Pin.vi"("Arduino Resource"=w1384, "Digital I/O Pin (0)"=u8 11, "Value (0)"=u8 1, "error in"=w1401) -> ("Arduino Resource"=w1408:T1, "error out"=w1409:errorcluster)  [unwired: 10 in]
        n318 = call <vilib>:"Digital Write Pin.vi"("Arduino Resource"=w1408, "Digital I/O Pin (0)"=u8 12, "Value (0)"=u8 0, "error in"=w1409) -> ("Arduino Resource"=w1403:T1, "error out"=w1402:errorcluster)  [unwired: 10 in]
        n319 = call <vilib>:"Digital Write Pin.vi"("Arduino Resource"=w1403, "Digital I/O Pin (0)"=u8 12, "Value (0)"=u8 1, "error in"=w1402) -> ("Arduino Resource"=w1412:T1, "error out"=w1413:errorcluster)  [unwired: 10 in]
        n320 = call <vilib>:"Digital Write Pin.vi"("Arduino Resource"=w1412, "Digital I/O Pin (0)"=u8 2, "Value (0)"=u8 1, "error in"=w1413) -> ("Arduino Resource"=w1414:T1, "error out"=w1302:errorcluster)  [unwired: 10 in]
        n321 = call <vilib>:"Digital Write Pin.vi"("Arduino Resource"=w1414, "Digital I/O Pin (0)"=u8 3, "Value (0)"=u8 1, "error in"=w1302) -> ("Arduino Resource"=w1415:T1, "error out"=w1303:errorcluster)  [unwired: 10 in]
        n322 = call <vilib>:"Digital Write Pin.vi"("Arduino Resource"=w1415, "Digital I/O Pin (0)"=u8 4, "Value (0)"=u8 1, "error in"=w1303) -> ("Arduino Resource"=w1416:T1, "error out"=w1304:errorcluster)  [unwired: 10 in]
        n323 = call <vilib>:"Digital Write Pin.vi"("Arduino Resource"=w1416, "Digital I/O Pin (0)"=u8 5, "Value (0)"=u8 1, "error in"=w1304) -> ("Arduino Resource"=w1417:T1, "error out"=w1305:errorcluster)  [unwired: 10 in]
        n324 = call <vilib>:"Digital Write Pin.vi"("Arduino Resource"=w1417, "Digital I/O Pin (0)"=u8 6, "Value (0)"=u8 1, "error in"=w1305) -> ("Arduino Resource"=w1418:T1, "error out"=w1306:errorcluster)  [unwired: 10 in]
        n325 = call <vilib>:"Digital Write Pin.vi"("Arduino Resource"=w1418, "Digital I/O Pin (0)"=u8 7, "Value (0)"=u8 1, "error in"=w1306) -> ("Arduino Resource"=w1419:T1, "error out"=w1307:errorcluster)  [unwired: 10 in]
        n326 = call <vilib>:"Digital Write Pin.vi"("Arduino Resource"=w1419, "Digital I/O Pin (0)"=u8 8, "Value (0)"=u8 1, "error in"=w1307) -> ("Arduino Resource"=w1420:T1, "error out"=w1308:errorcluster)  [unwired: 10 in]
        n327 = call <vilib>:"Digital Write Pin.vi"("Arduino Resource"=w1420, "Digital I/O Pin (0)"=u8 9, "Value (0)"=u8 1, "error in"=w1308) -> ("Arduino Resource"=w1421:T1, "error out"=w1309:errorcluster)  [unwired: 10 in]
        n328 = call <vilib>:"Digital Write Pin.vi"("Arduino Resource"=w1421, "Digital I/O Pin (0)"=u8 10, "Value (0)"=u8 1, "error in"=w1309) -> ("Arduino Resource"=w1422:T1, "error out"=w1310:errorcluster)  [unwired: 10 in]
        n329 = call <vilib>:"Digital Write Pin.vi"("Arduino Resource"=w1422, "Digital I/O Pin (0)"=u8 11, "Value (0)"=u8 0, "error in"=w1310) -> ("Arduino Resource"=w1317:T1, "error out"=w1318:errorcluster)  [unwired: 10 in]
        n330 = call <vilib>:"Digital Write Pin.vi"("Arduino Resource"=w1317, "Digital I/O Pin (0)"=u8 12, "Value (0)"=u8 0, "error in"=w1318) -> ("Arduino Resource"=w1312:T1, "error out"=w1311:errorcluster)  [unwired: 10 in]
        n331 = call <vilib>:"Digital Write Pin.vi"("Arduino Resource"=w1312, "Digital I/O Pin (0)"=u8 12, "Value (0)"=u8 1, "error in"=w1311) -> ("Arduino Resource"=w1281:T1, "error out"=w1280:errorcluster)  [unwired: 10 in]
      }
      frame 0, Default {
        n332 = call <vilib>:"Digital Write Pin.vi"("Arduino Resource"=w1426, "Digital I/O Pin (0)"=u8 2, "Value (0)"=u8 1, "error in"=w1425) -> ("Arduino Resource"=w1501:T1, "error out"=w1500:errorcluster)  [unwired: 10 in]
        n333 = call <vilib>:"Digital Write Pin.vi"("Arduino Resource"=w1501, "Digital I/O Pin (0)"=u8 3, "Value (0)"=u8 1, "error in"=w1500) -> ("Arduino Resource"=w1499:T1, "error out"=w1498:errorcluster)  [unwired: 10 in]
        n334 = call <vilib>:"Digital Write Pin.vi"("Arduino Resource"=w1499, "Digital I/O Pin (0)"=u8 4, "Value (0)"=u8 1, "error in"=w1498) -> ("Arduino Resource"=w1497:T1, "error out"=w1496:errorcluster)  [unwired: 10 in]
        n335 = call <vilib>:"Digital Write Pin.vi"("Arduino Resource"=w1497, "Digital I/O Pin (0)"=u8 5, "Value (0)"=u8 1, "error in"=w1496) -> ("Arduino Resource"=w1495:T1, "error out"=w1494:errorcluster)  [unwired: 10 in]
        n336 = call <vilib>:"Digital Write Pin.vi"("Arduino Resource"=w1495, "Digital I/O Pin (0)"=u8 6, "Value (0)"=u8 1, "error in"=w1494) -> ("Arduino Resource"=w1493:T1, "error out"=w1492:errorcluster)  [unwired: 10 in]
        n337 = call <vilib>:"Digital Write Pin.vi"("Arduino Resource"=w1493, "Digital I/O Pin (0)"=u8 7, "Value (0)"=u8 1, "error in"=w1492) -> ("Arduino Resource"=w1491:T1, "error out"=w1490:errorcluster)  [unwired: 10 in]
        n338 = call <vilib>:"Digital Write Pin.vi"("Arduino Resource"=w1491, "Digital I/O Pin (0)"=u8 8, "Value (0)"=u8 1, "error in"=w1490) -> ("Arduino Resource"=w1489:T1, "error out"=w1488:errorcluster)  [unwired: 10 in]
        n339 = call <vilib>:"Digital Write Pin.vi"("Arduino Resource"=w1489, "Digital I/O Pin (0)"=u8 9, "Value (0)"=u8 1, "error in"=w1488) -> ("Arduino Resource"=w1487:T1, "error out"=w1486:errorcluster)  [unwired: 10 in]
        n340 = call <vilib>:"Digital Write Pin.vi"("Arduino Resource"=w1487, "Digital I/O Pin (0)"=u8 10, "Value (0)"=u8 0, "error in"=w1486) -> ("Arduino Resource"=w1485:T1, "error out"=w1484:errorcluster)  [unwired: 10 in]
        n341 = call <vilib>:"Digital Write Pin.vi"("Arduino Resource"=w1485, "Digital I/O Pin (0)"=u8 11, "Value (0)"=u8 0, "error in"=w1484) -> ("Arduino Resource"=w1502:T1, "error out"=w1503:errorcluster)  [unwired: 10 in]
        n342 = call <vilib>:"Digital Write Pin.vi"("Arduino Resource"=w1502, "Digital I/O Pin (0)"=u8 12, "Value (0)"=u8 0, "error in"=w1503) -> ("Arduino Resource"=w1505:T1, "error out"=w1504:errorcluster)  [unwired: 10 in]
        n343 = call <vilib>:"Digital Write Pin.vi"("Arduino Resource"=w1505, "Digital I/O Pin (0)"=u8 12, "Value (0)"=u8 1, "error in"=w1504) -> ("Arduino Resource"=w1556:T1, "error out"=w1557:errorcluster)  [unwired: 10 in]
        n344 = call <vilib>:"Digital Write Pin.vi"("Arduino Resource"=w1556, "Digital I/O Pin (0)"=u8 2, "Value (0)"=u8 1, "error in"=w1557) -> ("Arduino Resource"=w1538:T1, "error out"=w1539:errorcluster)  [unwired: 10 in]
        n345 = call <vilib>:"Digital Write Pin.vi"("Arduino Resource"=w1538, "Digital I/O Pin (0)"=u8 3, "Value (0)"=u8 1, "error in"=w1539) -> ("Arduino Resource"=w1537:T1, "error out"=w1540:errorcluster)  [unwired: 10 in]
        n346 = call <vilib>:"Digital Write Pin.vi"("Arduino Resource"=w1537, "Digital I/O Pin (0)"=u8 4, "Value (0)"=u8 1, "error in"=w1540) -> ("Arduino Resource"=w1536:T1, "error out"=w1541:errorcluster)  [unwired: 10 in]
        n347 = call <vilib>:"Digital Write Pin.vi"("Arduino Resource"=w1536, "Digital I/O Pin (0)"=u8 5, "Value (0)"=u8 1, "error in"=w1541) -> ("Arduino Resource"=w1535:T1, "error out"=w1542:errorcluster)  [unwired: 10 in]
        n348 = call <vilib>:"Digital Write Pin.vi"("Arduino Resource"=w1535, "Digital I/O Pin (0)"=u8 6, "Value (0)"=u8 1, "error in"=w1542) -> ("Arduino Resource"=w1534:T1, "error out"=w1543:errorcluster)  [unwired: 10 in]
        n349 = call <vilib>:"Digital Write Pin.vi"("Arduino Resource"=w1534, "Digital I/O Pin (0)"=u8 7, "Value (0)"=u8 1, "error in"=w1543) -> ("Arduino Resource"=w1533:T1, "error out"=w1544:errorcluster)  [unwired: 10 in]
        n350 = call <vilib>:"Digital Write Pin.vi"("Arduino Resource"=w1533, "Digital I/O Pin (0)"=u8 8, "Value (0)"=u8 1, "error in"=w1544) -> ("Arduino Resource"=w1532:T1, "error out"=w1545:errorcluster)  [unwired: 10 in]
        n351 = call <vilib>:"Digital Write Pin.vi"("Arduino Resource"=w1532, "Digital I/O Pin (0)"=u8 9, "Value (0)"=u8 1, "error in"=w1545) -> ("Arduino Resource"=w1531:T1, "error out"=w1546:errorcluster)  [unwired: 10 in]
        n352 = call <vilib>:"Digital Write Pin.vi"("Arduino Resource"=w1531, "Digital I/O Pin (0)"=u8 10, "Value (0)"=u8 0, "error in"=w1546) -> ("Arduino Resource"=w1530:T1, "error out"=w1547:errorcluster)  [unwired: 10 in]
        n353 = call <vilib>:"Digital Write Pin.vi"("Arduino Resource"=w1530, "Digital I/O Pin (0)"=u8 11, "Value (0)"=u8 1, "error in"=w1547) -> ("Arduino Resource"=w1554:T1, "error out"=w1555:errorcluster)  [unwired: 10 in]
        n354 = call <vilib>:"Digital Write Pin.vi"("Arduino Resource"=w1554, "Digital I/O Pin (0)"=u8 12, "Value (0)"=u8 0, "error in"=w1555) -> ("Arduino Resource"=w1549:T1, "error out"=w1548:errorcluster)  [unwired: 10 in]
        n355 = call <vilib>:"Digital Write Pin.vi"("Arduino Resource"=w1549, "Digital I/O Pin (0)"=u8 12, "Value (0)"=u8 1, "error in"=w1548) -> ("Arduino Resource"=w1558:T1, "error out"=w1559:errorcluster)  [unwired: 10 in]
        n356 = call <vilib>:"Digital Write Pin.vi"("Arduino Resource"=w1558, "Digital I/O Pin (0)"=u8 2, "Value (0)"=u8 1, "error in"=w1559) -> ("Arduino Resource"=w1560:T1, "error out"=w1448:errorcluster)  [unwired: 10 in]
        n357 = call <vilib>:"Digital Write Pin.vi"("Arduino Resource"=w1560, "Digital I/O Pin (0)"=u8 3, "Value (0)"=u8 1, "error in"=w1448) -> ("Arduino Resource"=w1561:T1, "error out"=w1449:errorcluster)  [unwired: 10 in]
        n358 = call <vilib>:"Digital Write Pin.vi"("Arduino Resource"=w1561, "Digital I/O Pin (0)"=u8 4, "Value (0)"=u8 1, "error in"=w1449) -> ("Arduino Resource"=w1562:T1, "error out"=w1450:errorcluster)  [unwired: 10 in]
        n359 = call <vilib>:"Digital Write Pin.vi"("Arduino Resource"=w1562, "Digital I/O Pin (0)"=u8 5, "Value (0)"=u8 1, "error in"=w1450) -> ("Arduino Resource"=w1563:T1, "error out"=w1451:errorcluster)  [unwired: 10 in]
        n360 = call <vilib>:"Digital Write Pin.vi"("Arduino Resource"=w1563, "Digital I/O Pin (0)"=u8 6, "Value (0)"=u8 1, "error in"=w1451) -> ("Arduino Resource"=w1564:T1, "error out"=w1452:errorcluster)  [unwired: 10 in]
        n361 = call <vilib>:"Digital Write Pin.vi"("Arduino Resource"=w1564, "Digital I/O Pin (0)"=u8 7, "Value (0)"=u8 1, "error in"=w1452) -> ("Arduino Resource"=w1565:T1, "error out"=w1453:errorcluster)  [unwired: 10 in]
        n362 = call <vilib>:"Digital Write Pin.vi"("Arduino Resource"=w1565, "Digital I/O Pin (0)"=u8 8, "Value (0)"=u8 1, "error in"=w1453) -> ("Arduino Resource"=w1566:T1, "error out"=w1454:errorcluster)  [unwired: 10 in]
        n363 = call <vilib>:"Digital Write Pin.vi"("Arduino Resource"=w1566, "Digital I/O Pin (0)"=u8 9, "Value (0)"=u8 1, "error in"=w1454) -> ("Arduino Resource"=w1567:T1, "error out"=w1455:errorcluster)  [unwired: 10 in]
        n364 = call <vilib>:"Digital Write Pin.vi"("Arduino Resource"=w1567, "Digital I/O Pin (0)"=u8 10, "Value (0)"=u8 1, "error in"=w1455) -> ("Arduino Resource"=w1568:T1, "error out"=w1456:errorcluster)  [unwired: 10 in]
        n365 = call <vilib>:"Digital Write Pin.vi"("Arduino Resource"=w1568, "Digital I/O Pin (0)"=u8 11, "Value (0)"=u8 0, "error in"=w1456) -> ("Arduino Resource"=w1463:T1, "error out"=w1464:errorcluster)  [unwired: 10 in]
        n366 = call <vilib>:"Digital Write Pin.vi"("Arduino Resource"=w1463, "Digital I/O Pin (0)"=u8 12, "Value (0)"=u8 0, "error in"=w1464) -> ("Arduino Resource"=w1458:T1, "error out"=w1457:errorcluster)  [unwired: 10 in]
        n367 = call <vilib>:"Digital Write Pin.vi"("Arduino Resource"=w1458, "Digital I/O Pin (0)"=u8 12, "Value (0)"=u8 1, "error in"=w1457) -> ("Arduino Resource"=w1424:T1, "error out"=w1423:errorcluster)  [unwired: 10 in]
      }
    }
    n368 = Add(x=w79, y=w74) -> (x+y=w78:dbl)
    n369 = Greater Or Equal?(x=w78, y=50) -> (x >= y?=w91:bool)
    n370 = Select(t=0, s=w91, f=w78) -> (s? t:f=w82:dbl)
    n371 = Select(t=0, s="OK Button", f=w82) -> (s? t:f=w80:dbl)
    n372 = feedback-in #1(w80) -> ()
  }
  n373 = call <vilib>:"Close.vi"("Arduino Resource"=w2, "error in"=w3) -> ("error out"=w1:errorcluster)  [unwired: 13 in]
  n374 = call <vilib>:"Simple Error Handler.vi"("error in (no error)"=w1) -> ()  [unwired: 4 in, 5 out]
